vi "BaTS_(Singles).vi"() -> ()   [LabVIEW 2009]
uses:
  <vilib>/Utility/file.llb/Read From Spreadsheet File (DBL).vi
  <vilib>/Utility/miscctls.llb/LVPositionTypeDef.ctl
  <vilib>/Utility/file.llb/Write To Spreadsheet File (I64).vi
  <vilib>/vision/NI_Vision_Development_Module.lvlib
panel:
  out "framesPerSecond":u32
  out "serve to point":dbl[](array[numeric])
  in  "Word._Application":refnum<k7>
  out "p2y":dbl[](array[numeric])
  out "p1y":dbl[](array[numeric])
  out "point frames":dbl[](array[numeric])
  out "service frames":dbl[](array[numeric])
  out "comp_p1 2":dbl[](array[numeric])
  out "comp_p2 2":dbl[](array[numeric])
  out "comp_p2":dbl[](array[numeric])
  out "comp_p1":dbl[](array[numeric])
  out "game":i32[][](array[numeric])
  out "save2_data":dbl[][](array[numeric])
  out "save1_data":dbl[][](array[numeric])
  out "save2":i32[][](array[numeric])
  out "save1":i32[][](array[numeric])
  out "filedata in":dbl[][](array[numeric]) format="%0.3f"
  out "edited\nevents":dbl[][](array[numeric])
  out "edited to play":dbl[](array[numeric])
  out "P2 position":bool
  out "P1 position":bool
  out "p2code":i32
  out "p1code":i32
  out "frames":dbl[](array[numeric])
  out "Events":bool[](array[boolean])
  out "coded data":dbl[][](array[numeric])
  out "frame data":dbl[][](array[numeric])
  out "Score":dbl[][](array[numeric])
  out "OH":bool[](array[boolean])
  out "BH":bool[](array[boolean])
  out "FH":bool[](array[boolean])
  in  "stop":bool
  in  "Tab Control":enum32{"Coding", "Display"}(tab)
  in  "Drag control":u32(slide) min=400 max=3000 scale=0.0..37378.0
  in  "UNDO":bool
  out "Last coded":i32
  in  "Progress...":i32(slide) min=400 max=3000 scale=0.0..36584.0
  in  "1":bool
  in  "E2":bool
  in  "E1":bool
  in  "P2":i32
  in  "W2":bool
  in  "W1":bool
  in  "P1":i32
  in  "Pause 2":bool
  in  "F_Fr":bool
  in  "S_Fr":bool
  out "Video":T1(plugin-control)
  in  "START":bool
  in  "Video file":path caption="Open AVI file"
  in  "Save data":path caption="Save data to file"
  in  "Start Coding":bool
  out "F_frame":u32
  out "S_frame":u32
  in  "playback speed":dbl(slide) step=0.25 scale=0.25..2.0
  in  "fast forward":bool
  in  "TL 2":bool
  in  "BR 2":bool
  in  "BL 2":bool
  in  "BM 2":bool
  in  "CR  2":bool
  in  "CM 2":bool
  in  "CL 2":bool
  in  "TR 2":bool
  in  "TM 2":bool
  in  "TL 3":bool
  in  "BR 3":bool
  in  "BL 3":bool
  in  "BM 3":bool
  in  "CR  3":bool
  in  "CM 3":bool
  in  "CL 3":bool
  in  "TR 3":bool
  in  "TM 3":bool
  in  "Pause 1":bool
  out "coding":i32[][](array[numeric])
  in  "1 6":bool
  in  "2 6":bool
  in  "3 6":bool
  in  "4 6":bool
  in  "5 6":bool
  in  "6 6":bool
  in  "7 6":bool
  in  "8 6":bool
  in  "1 5":bool
  in  "2 5":bool
  in  "3 5":bool
  in  "4 5":bool
  in  "5 5":bool
  in  "6 5":bool
  in  "7 5":bool
  in  "8 5":bool
  in  "8 3":bool
  in  "7 3":bool
  in  "6 3":bool
  in  "5 3":bool
  in  "4 3":bool
  in  "3 3":bool
  in  "2 3":bool
  in  "1 3":bool
  in  "8 4":bool
  in  "7 4":bool
  in  "6 4":bool
  in  "5 4":bool
  in  "4 4":bool
  in  "3 4":bool
  in  "2 4":bool
  in  "1 4":bool
  in  "1 2":bool
  in  "2 2":bool
  in  "3 2":bool
  in  "4 2":bool
  in  "5 2":bool
  in  "6 2":bool
  in  "7 2":bool
  in  "8 2":bool
  in  "5":bool
  in  "6":bool
  in  "7":bool
  in  "8":bool
  in  "1":bool
  in  "2":bool
  in  "3":bool
  in  "4":bool
  in  "S2":bool
  in  "S1":bool
  in  "2":bool
  in  "3":bool
  in  "4":bool
  in  "Pause 3":bool
  in  "court":bool
  in  "Stop and save":bool
  out "Numeric":dbl format="%<%H:%M:%S>t"
  in  "play back":i32(slide)=1 min=0 max=1212 scale=0.0..1212.0
  out "DISP":T1(plugin-control)
  in  "Vid file":path caption="Open AVI file"
  in  "Data file":path caption="Read data from"
  in  "Tab Control 2":enum32{"Edit ", "Data Display", "Momentum"}(tab)
  in  "shots":u8(slide)=2 scale=0.0..5.0
  in  "point 2":bool
  in  "Rally":bool
  in  "Write VI":path caption="Write to AVI file"
  in  "before":u8(slide)=2 scale=5.0..0.0
  in  "Playback Speed":dbl(slide)=1.0 min=0.25 max=30.0 step=0.25 scale=0.25..2.0
  in  "pause":bool
  in  "stop 2":bool
  in  "Playback\nscore":bool
  in  "P2 score":dbl
  in  "P1 score":dbl
  in  "error":bool
  in  "winner":bool
  in  "point 1":bool
  in  "player1":bool
  in  "player2":bool
  in  "1 7":bool
  in  "service2":bool
  in  "service1":bool
  in  "2 7":bool
  in  "3 7":bool
  in  "4 7":bool
  in  "TL":bool
  in  "BR":bool
  in  "BL":bool
  in  "BM":bool
  in  "CR":bool
  in  "CM":bool
  in  "CL":bool
  in  "TR":bool
  in  "TM":bool
  in  "FH 2":bool
  in  "BH 2":bool
  in  "ST":bool
  in  "CR 2":bool
  in  "lob":bool
  in  "clear":bool
  in  "drive":bool
  in  "smash":bool
  in  "defense":bool
  in  "chop":bool
  in  "drop":bool
  in  "net":bool
  in  "OH 2":bool
  in  "Play":bool
  in  "after":u8(slide)=2 scale=0.0..5.0
  in  "write file":bool
  out "Search events":i32(slide) caption="Scaning(events)..." min=400 max=3000 scale=0.0..903.0
  out "Search score":i32(slide) caption="Searching(score)..." min=400 max=3000 scale=0.0..867.0
  out "writing":i32(slide) caption="Writing..." min=400 max=3000 scale=0.0..1212.0
  in  "3 shots":bool
  in  "Compare":bool
  in  "2":string(combo)="1"
  in  "1":string(combo)="1"
  in  "save2":string
  in  "save1":string
  in  "save2":bool
  in  "save1":bool
  in  "Percentage":bool
  in  "display\nselection":string(combo)="1"
  in  "To make white":enum32{""}(tab)
  out "player1 2":string[](array[string])
  out "player2 2":string[](array[string])
  out "P1graph":cluster{dbl[], "array":dbl[]}(graph)={[0.0, nan, 0.0, nan, 0.0, nan, 0.0, nan, 0.0, nan, 0.0, nan, 0.0, nan, 0.0, nan, 0.0], "array"=[1.0, 2.0, 3.0, 4.0, 5.0, 6.0, 7.0, 8.0, 9.0, 10.0, 11.0, 12.0, 13.0, 14.0, 15.0, 16.0, 17.0]}
  out "P2graph":cluster{dbl[], "array":dbl[]}(graph)={[0.0, nan, 0.0, nan, 0.0, nan, 0.0, nan, 0.0, nan, 0.0, nan, 0.0, nan, 0.0, nan, 0.0], "array"=[1.0, 2.0, 3.0, 4.0, 5.0, 6.0, 7.0, 8.0, 9.0, 10.0, 11.0, 12.0, 13.0, 14.0, 15.0, 16.0, 17.0]}
  out "W1/E1":string[](array[string])
  out "W2/E2":string[](array[string])
  out "W/E2":string[](array[string])=["Fore hand", "Back hand", "Over head", "", "Strainght", "Cross", "", "Lob", "Clear", "Drive", "Smash", "Defence", "Chop", "Drop", "Net"]
  out "W/E1":string[](array[string])=["Fore hand", "Back hand", "Over head", "", "Strainght", "Cross", "", "Lob", "Clear", "Drive", "Smash", "Defence", "Chop", "Drop", "Net"]
  out "player2_2":string[](array[string])
  out "player1_2":string[](array[string])
  out "Player 2":string[](array[string])=["Fore hand", "Back hand", "Over head", "", "Straight", "Cross", "", "Smash", "Defense", "Drive/Tap", "Lob", "Drop", "Chop", "Clear", "Net"]
  out "Player 2_2":string[](array[string])=["Fore hand", "Back hand", "Over head", "", "Strainght", "Cross", "", "Lob", "Clear", "Drive", "Smash", "Defence", "Chop", "Drop", "Net"]
  out "Player 1_2":string[](array[string])=["Fore hand", "Back hand", "Over head", "", "Strainght", "Cross", "", "Lob", "Clear", "Drive", "Smash", "Defence", "Chop", "Drop", "Net"]
  out "Player 1":string[](array[string])=["Fore hand", "Back hand", "Over head", "", "Straight", "Cross", "", "Smash", "Defense", "Drive/Tap", "Lob", "Drop", "Chop", "Clear", "Net"]
  out "p2 17":string
  out "p2 16":string
  out "p2 11":string
  out "p2 10":string
  out "p2 9":string
  out "p2 14":string
  out "p2 13":string
  out "p2 12":string
  out "p2 15":string
  out "p1 5":string
  out "p1 7":string
  out "p1 6":string
  out "p1 4":string
  out "p1 1":string
  out "p1 3":string
  out "p1 2":string
  out "p1 8":string
  out "p1 9":string
  in  "to make white 2":enum32{""}(tab)
  out "Shortest rally length(sec)":dbl format="%#_3g"
  out "Longest rally length(sec)":dbl format="%#_3g"
  out "momentum graph":cluster{dbl[], dbl[]}[](graph)
  out "Score":dbl[](array[numeric])
  out "Average rally length(sec)":dbl format="%#_3g"
  out "Rally length(sec)":dbl format="%#_3g"
  in  "edit video":bool
  in  "REPORT":bool
  # "Strategic Analysis Tool for Badminton"
  # "Forehand"
  # "Backhand"
  # "Overhead"
  # "Position"
  # "Straight"
  # "Cross"
  # "Straight"
  # "Cross"
  # "Straight"
  # "Cross"
  # "Smash"
  # "Defence"
  # "Drive/Tap"
  # "Lob"
  # "Drop"
  # "Chop"
  # "Player 2\n\nPlayer 1"
  # "Player 1\n\nPlayer 2"
  # "Clear"
  # "Net"
  # "Score"
  # "© 2012 National Sports Institute of Malaysia All Rights Reserved"
  # "© 2012 National Sports Institute of Malaysia All Rights Reserved"
  # "Shots to Playback"
  # "Score"
  # "Player"
  # "Position"
  # "Special Events"
  # "Playback interval (s)"
  # "to"
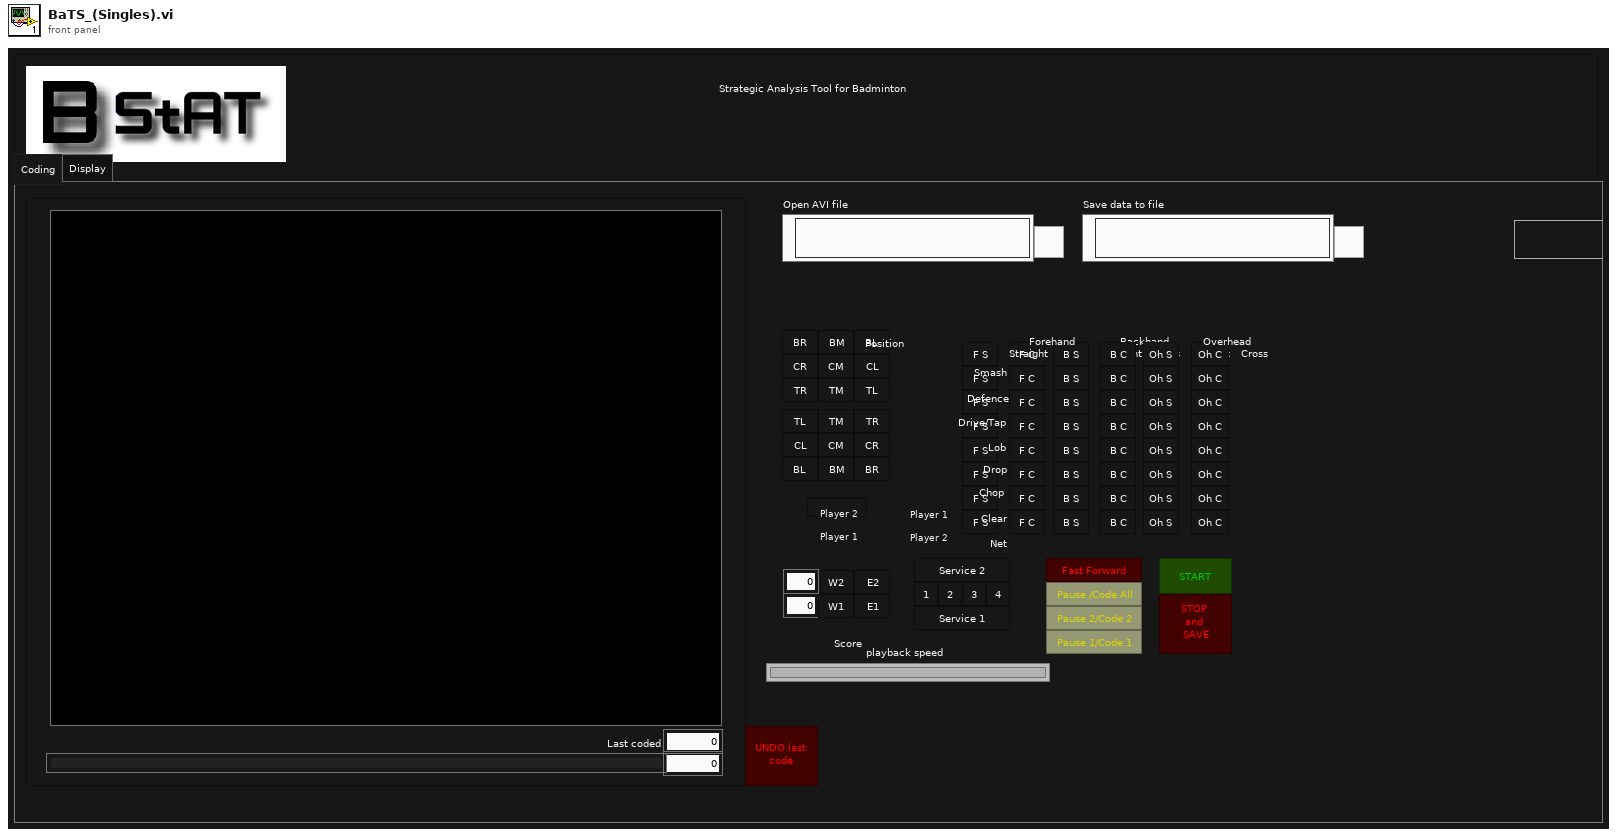
[diagram p1: front panel]
types:
  T1 = typedef "IMAQ Image.ctl" = refnum<image>
  T2 = enum16{"open", "replace", "create", "open or create", "replace or create", "replace or create with confirmation"}
  T3 = typedef "LVPositionTypeDef.ctl" = cluster{"Left":i32, "Top":i32}
  T4 = typedef "Image Type" = u32
  T5 = typedef "AviRefnum.ctl" = refnum<k1>
  T6 = cluster{"width":u32, "height":u32, "framesPerSecond":u32, "compressionFilter":string, "hasData":bool}
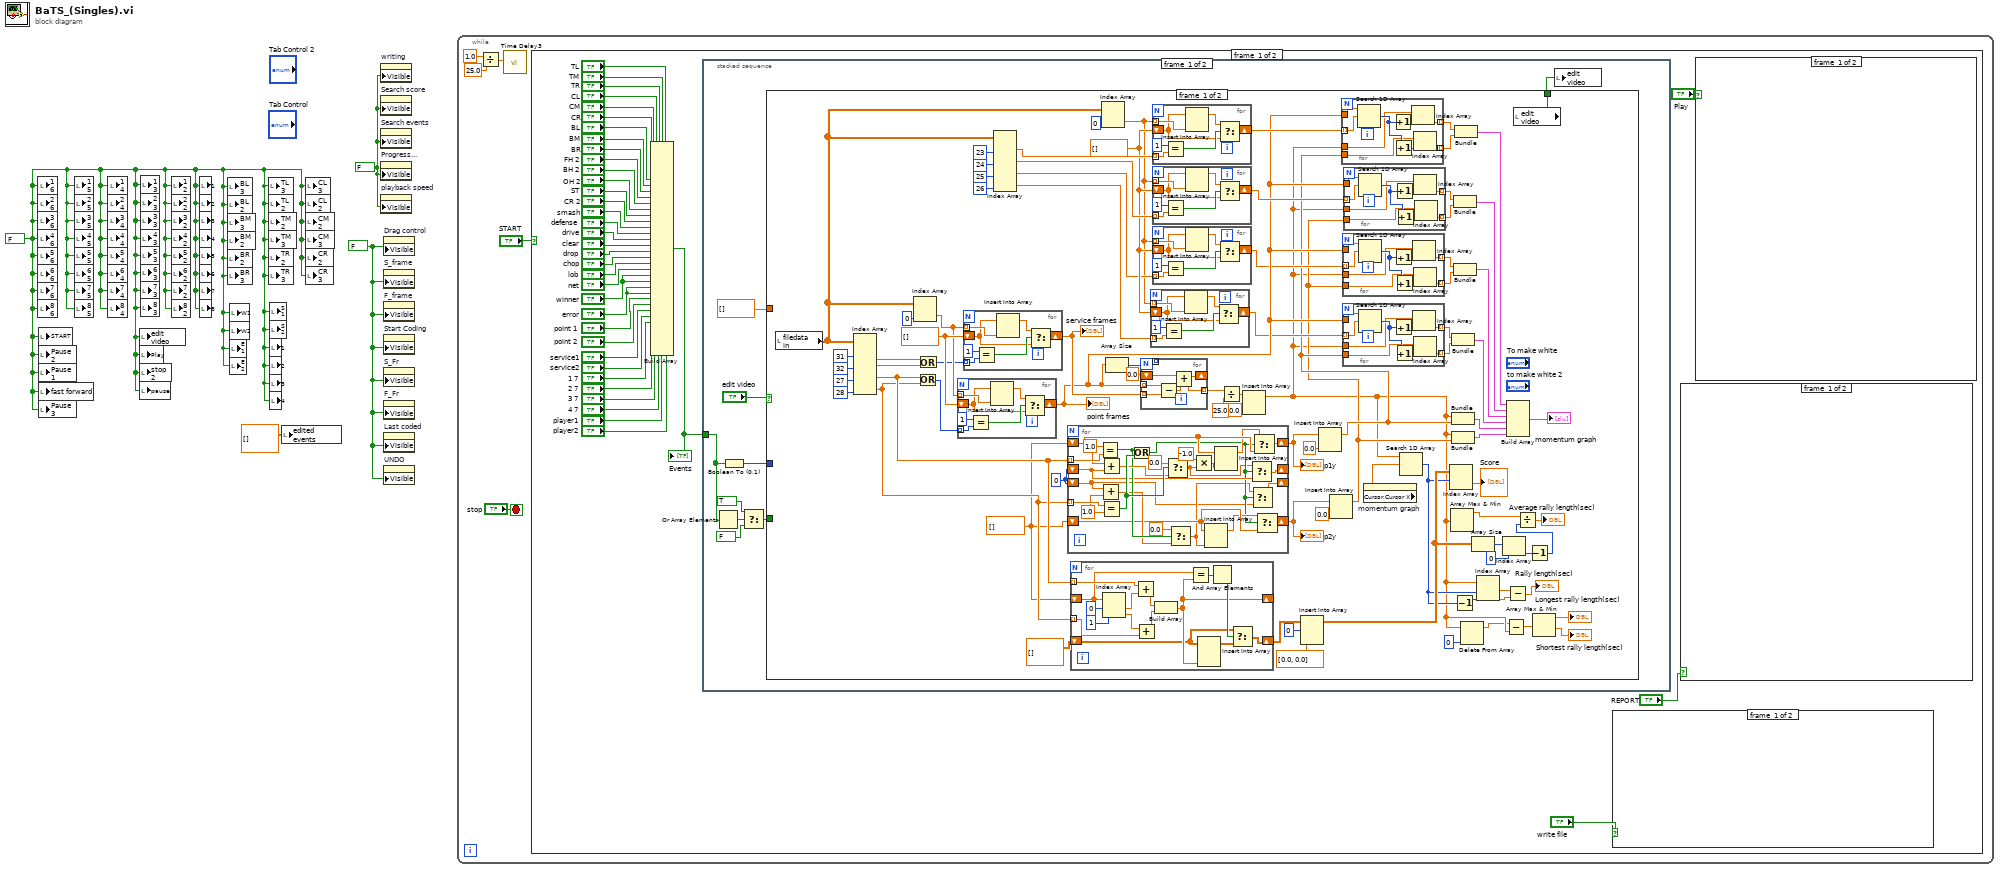
[diagram p0: block diagram]
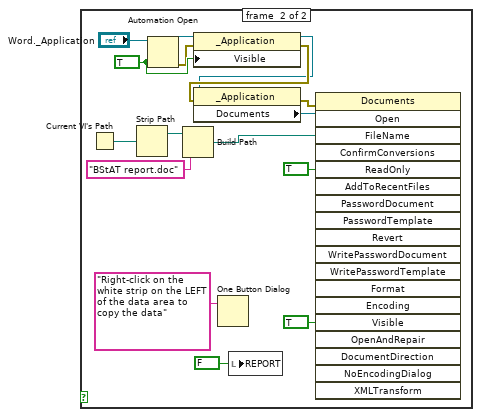
[diagram p2: hidden frame]
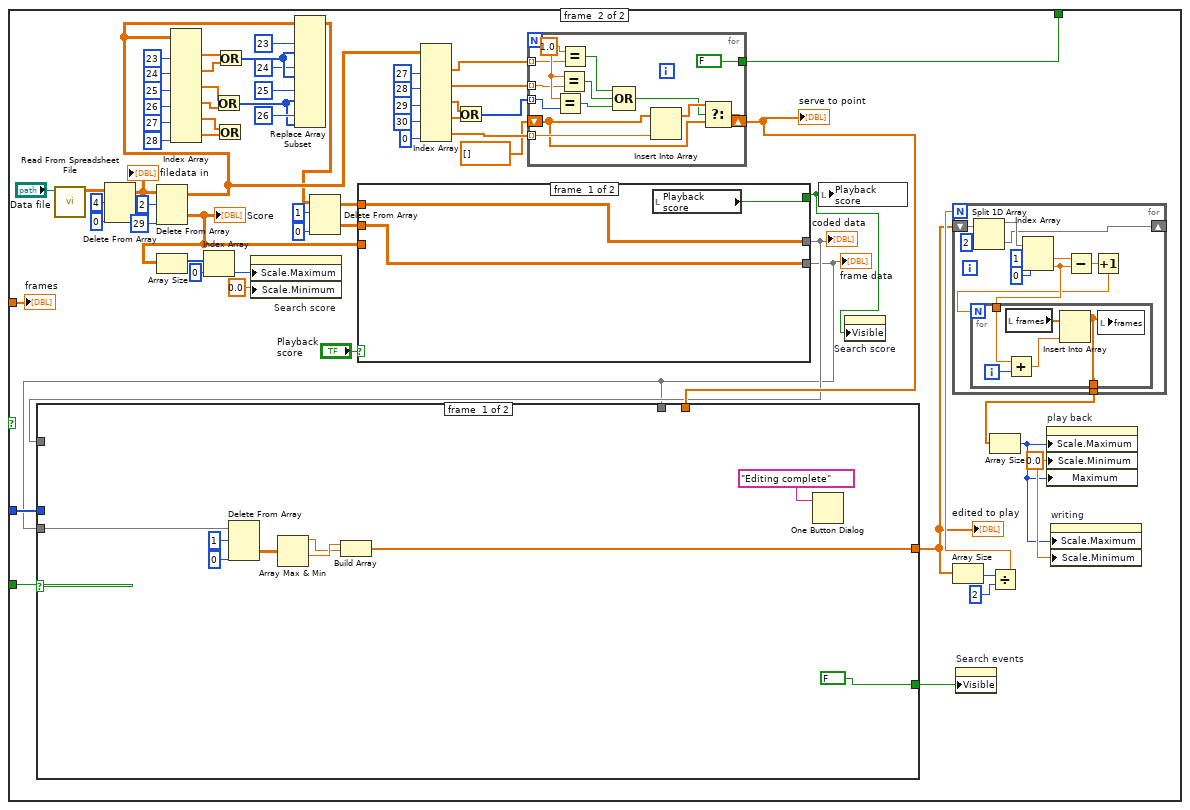
[diagram p3: hidden frame]
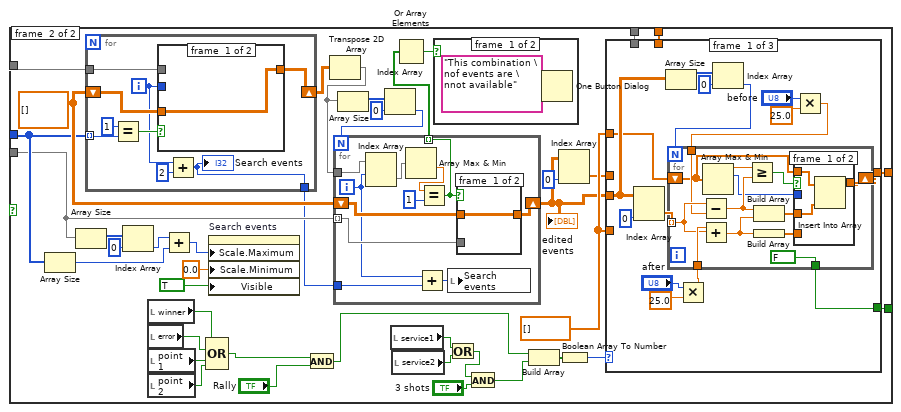
[diagram p4: hidden frame]
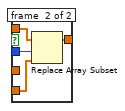
[diagram p5: hidden frame]
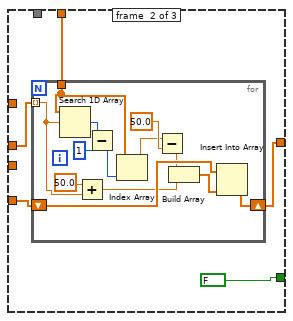
[diagram p6: hidden frame]
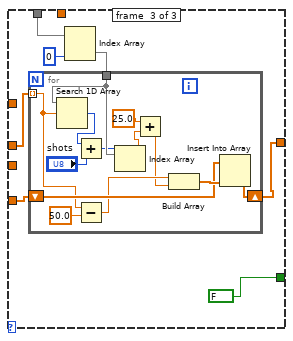
[diagram p7: hidden frame]
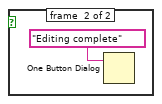
[diagram p8: hidden frame]
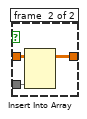
[diagram p9: hidden frame]
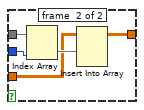
[diagram p10: hidden frame]
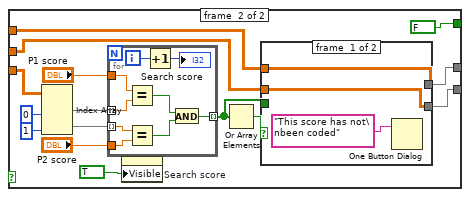
[diagram p11: hidden frame]
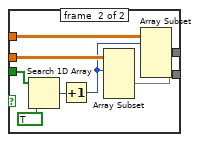
[diagram p12: hidden frame]
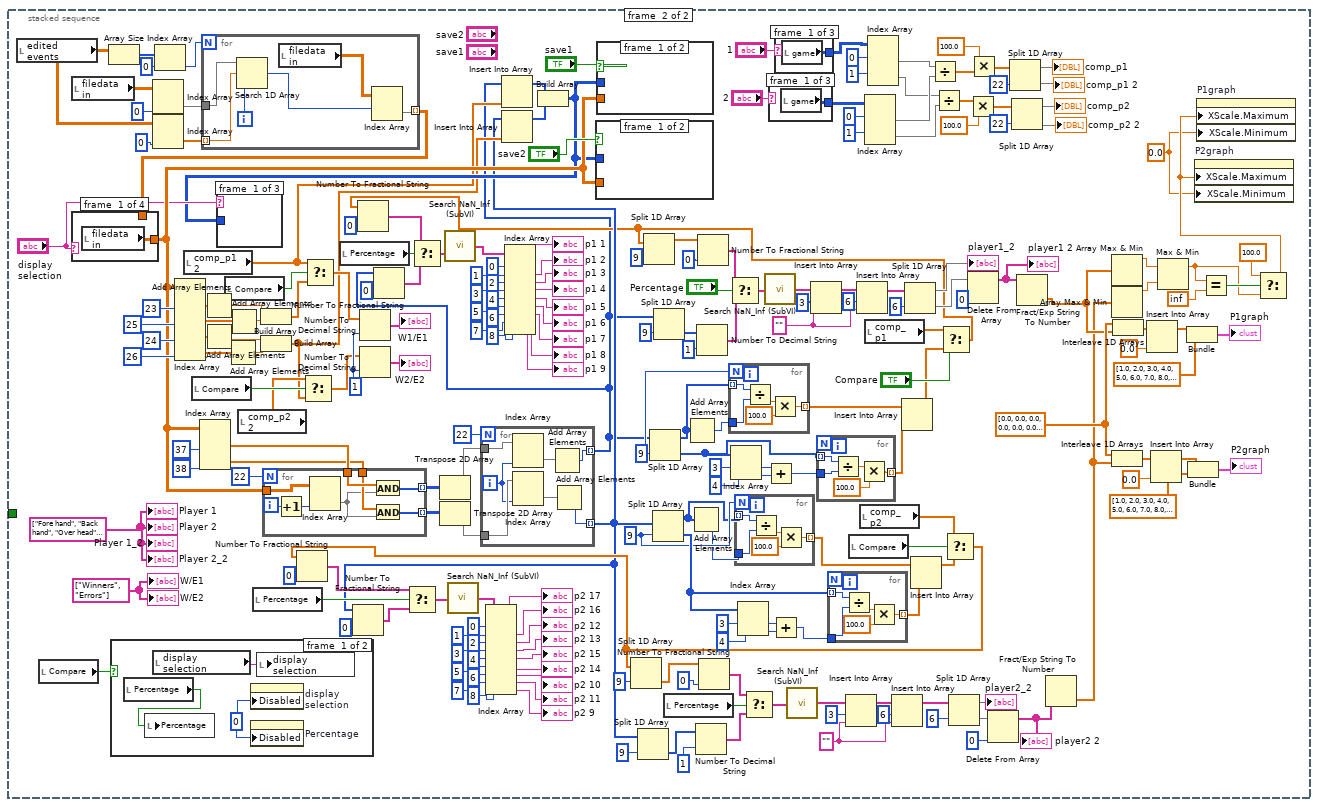
[diagram p13: hidden frame]
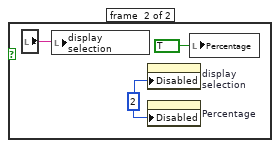
[diagram p14: hidden frame]
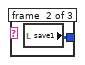
[diagram p15: hidden frame]
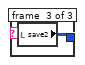
[diagram p16: hidden frame]
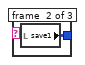
[diagram p17: hidden frame]
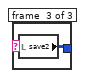
[diagram p18: hidden frame]
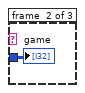
[diagram p19: hidden frame]
diagram:
  w2 = FALSE ("4 6")
  w1 = FALSE ("Visible")
  w3 = FALSE ("Visible")
  n1 = local write "1 6"(w2) -> ()
  n2 = local write "2 6"(w2) -> ()
  n3 = local write "3 6"(w2) -> ()
  n4 = local write "4 6"(w2) -> ()
  n5 = local write "5 6"(w2) -> ()
  n6 = local write "6 6"(w2) -> ()
  n7 = local write "7 6"(w2) -> ()
  n8 = local write "8 6"(w2) -> ()
  n9 = local write "START"(w2) -> ()
  n10 = local write "Pause 2"(w2) -> ()
  n11 = local write "Pause 1"(w2) -> ()
  n12 = local write "fast forward"(w2) -> ()
  n13 = local write "Pause 3"(w2) -> ()
  n14 = local write "1 5"(w2) -> ()
  n15 = local write "2 5"(w2) -> ()
  n16 = local write "3 5"(w2) -> ()
  n17 = local write "4 5"(w2) -> ()
  n18 = local write "5 5"(w2) -> ()
  n19 = local write "6 5"(w2) -> ()
  n20 = local write "7 5"(w2) -> ()
  n21 = local write "8 5"(w2) -> ()
  n22 = local write "1 4"(w2) -> ()
  n23 = local write "2 4"(w2) -> ()
  n24 = local write "3 4"(w2) -> ()
  n25 = local write "4 4"(w2) -> ()
  n26 = local write "5 4"(w2) -> ()
  n27 = local write "6 4"(w2) -> ()
  n28 = local write "7 4"(w2) -> ()
  n29 = local write "8 4"(w2) -> ()
  n30 = local write "edit video"(w2) -> ()
  n31 = local write "Play"(w2) -> ()
  n32 = local write "stop 2"(w2) -> ()
  n33 = local write "pause"(w2) -> ()
  n34 = local write "1 3"(w2) -> ()
  n35 = local write "2 3"(w2) -> ()
  n36 = local write "3 3"(w2) -> ()
  n37 = local write "4 3"(w2) -> ()
  n38 = local write "5 3"(w2) -> ()
  n39 = local write "6 3"(w2) -> ()
  n40 = local write "7 3"(w2) -> ()
  n41 = local write "8 3"(w2) -> ()
  n42 = local write "1 2"(w2) -> ()
  n43 = local write "2 2"(w2) -> ()
  n44 = local write "3 2"(w2) -> ()
  n45 = local write "4 2"(w2) -> ()
  n46 = local write "5 2"(w2) -> ()
  n47 = local write "6 2"(w2) -> ()
  n48 = local write "7 2"(w2) -> ()
  n49 = local write "8 2"(w2) -> ()
  n50 = local write "1"(w2) -> ()
  n51 = local write "2"(w2) -> ()
  n52 = local write "3"(w2) -> ()
  n53 = local write "4"(w2) -> ()
  n54 = local write "5"(w2) -> ()
  n55 = local write "6"(w2) -> ()
  n56 = local write "7"(w2) -> ()
  n57 = local write "8"(w2) -> ()
  n58 = local write "BL 3"(w2) -> ()
  n59 = local write "BL 2"(w2) -> ()
  n60 = local write "BM 3"(w2) -> ()
  n61 = local write "BM 2"(w2) -> ()
  n62 = local write "BR 2"(w2) -> ()
  n63 = local write "BR 3"(w2) -> ()
  n64 = local write "W1"(w2) -> ()
  n65 = local write "W2"(w2) -> ()
  n66 = local write "E1"(w2) -> ()
  n67 = local write "E2"(w2) -> ()
  n68 = local write "TL 3"(w2) -> ()
  n69 = local write "TL 2"(w2) -> ()
  n70 = local write "TM 2"(w2) -> ()
  n71 = local write "TM 3"(w2) -> ()
  n72 = local write "TR 2"(w2) -> ()
  n73 = local write "TR 3"(w2) -> ()
  n74 = local write "S1"(w2) -> ()
  n75 = local write "S2"(w2) -> ()
  n76 = local write "1"(w2) -> ()
  n77 = local write "2"(w2) -> ()
  n78 = local write "3"(w2) -> ()
  n79 = local write "4"(w2) -> ()
  n80 = local write "edited\nevents"(dbl[][] []) -> ()
  n81 = local write "CL 3"(w2) -> ()
  n82 = local write "CL 2"(w2) -> ()
  n83 = local write "CM 2"(w2) -> ()
  n84 = local write "CM 3"(w2) -> ()
  n85 = local write "CR  2"(w2) -> ()
  n86 = local write "CR  3"(w2) -> ()
  n87 = property on="writing" class="Slide (strict)"("Visible"=w3) -> ()  [unwired: 2 in, 2 out]
  n88 = property on="Search score" class="Slide (strict)"("Visible"=w3) -> ()  [unwired: 2 in, 2 out]
  n89 = property on="Search events" class="Slide (strict)"("Visible"=w3) -> ()  [unwired: 2 in, 2 out]
  n90 = property on="Progress..." class="Slide (strict)"("Visible"=w3) -> ()  [unwired: 2 in, 2 out]
  n91 = property on="playback speed" class="Slide (strict)"("Visible"=w3) -> ()  [unwired: 2 in, 2 out]
  n92 = property on="Drag control" class="Slide (strict)"("Visible"=w1) -> ()  [unwired: 2 in, 2 out]
  n93 = property on="S_frame" class="DigNum (strict)"("Visible"=w1) -> ()  [unwired: 2 in, 2 out]
  n94 = property on="F_frame" class="DigNum (strict)"("Visible"=w1) -> ()  [unwired: 2 in, 2 out]
  n95 = property on="Start Coding" class="Bool (strict)"("Visible"=w1) -> ()  [unwired: 2 in, 2 out]
  n96 = property on="S_Fr" class="Bool (strict)"("Visible"=w1) -> ()  [unwired: 2 in, 2 out]
  n97 = property on="F_Fr" class="Bool (strict)"("Visible"=w1) -> ()  [unwired: 2 in, 2 out]
  n98 = property on="Last coded" class="DigNum (strict)"("Visible"=w1) -> ()  [unwired: 2 in, 2 out]
  n99 = property on="UNDO" class="Bool (strict)"("Visible"=w1) -> ()  [unwired: 2 in, 2 out]
  n100 = while {
    stop <- "stop" stop-if-true
    n101 = Divide(x=1.0, y=25.0) -> (x/y=w5:dbl)
    n102 = call "Time Delay3"("Delay Time (s)"=w5) -> ()  [unwired: 10 in, 1 out]
    n103 = case shown="True" "START" {
      frame #0 {
        n104 = Build Array("TL", "TM", "TR", "CL", "CM", "CR", "BL", "BM", "BR", "FH 2", "BH 2", "OH 2", "ST", "CR 2", "smash", "defense", "drive", "clear", "drop", "chop", "lob", "net", "winner", "winner", "error", "error", "point 1", "point 2", "service1", "service2", "1 7", "2 7", "3 7", "4 7", "player1", "player2") -> (w22:bool[])
        "Events" <- w22
        n105 = stacked-sequence {
          tunnel: w22 -> [w69 _]
          frame #0 {
            n106 = Or Array Elements(Boolean array=w69) -> (logical OR=w72:bool)
            n107 = Boolean To (0,1)(Boolean=w69) -> (0, 1=w68:i16[])
            n108 = Select(t=TRUE, s=w72, f=FALSE) -> (s? t:f=w67:bool)
            n109 = case shown="True" "edit video" {
              tunnel: [w157 w287] -> w65
              tunnel: w68 -> [_ w285]
              tunnel: w67 -> [_ w329]
              tunnel: dbl[] [] ("edited\nto play 3") -> [_ w327]
              frame #0 {
                w113 = dbl[] []
                w147 = 0.0 ("new element/subarray")
                w146 = 0.0 ("new element/subarray")
                w145 = 0.0 ("new element/subarray")
                w95 = dbl[] []
                w98 = 0 ("disabled index (col)")
                w138 = dbl[] []
                n110 = local read "filedata in"() -> (w114:dbl[][])
                n111 = Index Array(array=w114, index (col) #1=31 ("length"), index (col) #2=32 ("disabled index (col)"), index (col) #3=27 ("index (col)"), index (col) #4=28 ("index (col)")) -> (element #1=w130:dbl[], element #2=w131:dbl[], element #3=w97:dbl[], element #4=w96:dbl[])  [unwired: 4 in]
                n112 = Index Array(array=w114, index (col)=0 ("disabled index (col)")) -> (element=w137:dbl[])  [unwired: 1 in]
                n113 = Or(x=w97, y=w96) -> (x .or. y?=w136:i32[])
                n114 = Or(x=w130, y=w131) -> (x .or. y?=w133:i32[])
                n115 = for {
                  tunnel: w136 -> [w274] mode=indexing
                  tunnel: w137 -> [w270] mode=indexing
                  shift-right: [w269] -> w109
                  shift-left: w138 -> [w268]
                  n116 = Equal?(x=1, y=w274) -> (x = y?=w272:bool)
                  n117 = Insert Into Array(array=w268, new element=w270) -> (w271:dbl[])  [unwired: 1 in]
                  n118 = Select(t=w271, s=w272, f=w268) -> (s? t:f=w269:dbl[])
                }
                "point frames" <- w109
                n119 = for {
                  tunnel: w133 -> [w281] mode=indexing
                  tunnel: w137 -> [w277] mode=indexing
                  shift-right: [w276] -> w140
                  shift-left: w138 -> [w275]
                  n120 = Equal?(x=1, y=w281) -> (x = y?=w279:bool)
                  n121 = Insert Into Array(array=w275, new element=w277) -> (w278:dbl[])  [unwired: 1 in]
                  n122 = Select(t=w278, s=w279, f=w275) -> (s? t:f=w276:dbl[])
                }
                "service frames" <- w140
                n123 = Index Array(array=w114, index (col) #1=23 ("disabled index (col)"), index (col) #2=24 ("index (col)"), index (col) #3=25 ("index (col)"), index (col) #4=26 ("index (col)")) -> (element #1=w123:dbl[], element #2=w124:dbl[], element #3=w112:dbl[], element #4=w111:dbl[])  [unwired: 4 in]
                n124 = for {
                  shift-right: [w166] -> _
                  shift-left: w98 -> [w165]
                  shift-right: [w162] -> _
                  shift-left: w98 -> [w161]
                  shift-right: [w171] -> w93
                  shift-left: w95 -> [w170]
                  shift-right: [w177] -> w94
                  shift-left: w95 -> [w168]
                  tunnel: w96 -> [w174] mode=indexing
                  tunnel: w97 -> [w182] mode=indexing
                  w173 = 1.0 ("x")
                  w179 = 1.0 ("x")
                  n125 = Equal?(x=w179, y=w182) -> (x = y?=w175:bool)
                  n126 = Add(x=w161, y=w173) -> (x+y=w172:dbl)
                  n127 = Add(x=w179, y=w165) -> (x+y=w178:dbl)
                  n128 = Equal?(x=w174, y=w173) -> (x = y?=w181:bool)
                  n129 = Or(x=w175, y=w181) -> (x .or. y?=w164:bool)
                  n130 = Select(t=0.0, s=w181, f=w178) -> (s? t:f=w158:dbl)
                  n131 = Select(t=0.0, s=w175, f=w172) -> (s? t:f=w163:dbl)
                  n132 = Multiply(x=-1.0 ("y"), y=w158) -> (x*y=w160:dbl)
                  n133 = Insert Into Array(array=w168, new element=w163) -> (w167:dbl[])  [unwired: 1 in]
                  n134 = Insert Into Array(array=w170, new element=w160) -> (w169:dbl[])  [unwired: 1 in]
                  n135 = Select(t=w158, s=w164, f=w165) -> (s? t:f=w166:dbl)
                  n136 = Select(t=w163, s=w164, f=w161) -> (s? t:f=w162:dbl)
                  n137 = Select(t=w169, s=w164, f=w170) -> (s? t:f=w171:dbl[])
                  n138 = Select(t=w167, s=w164, f=w168) -> (s? t:f=w177:dbl[])
                }
                "p1y" <- w93
                "p2y" <- w94
                n139 = for {
                  tunnel: w97 -> [w258] mode=indexing
                  tunnel: w96 -> [w254] mode=indexing
                  shift-right: [w250] -> _
                  shift-left: w95 -> [w253]
                  shift-right: [w248] -> w152
                  shift-left: dbl[][] [] -> [w247]
                  n140 = Index Array(array=w253, index #1=0 ("index"), index #2=1 ("index")) -> (element #1=w259:dbl, element #2=w257:dbl)
                  n141 = Add(x=w258, y=w259) -> (x+y=w256:dbl)
                  n142 = Add(x=w257, y=w254) -> (x+y=w255:dbl)
                  n143 = Build Array(w256, w255) -> (w250:dbl[])
                  n144 = Equal?(x=w253, y=w250) -> (x = y?=w252:bool[])
                  n145 = Insert Into Array(array=w247, new element=w250) -> (w249:dbl[][])  [unwired: 2 in]
                  n146 = And Array Elements(Boolean array=w252) -> (logical AND=w251:bool)
                  n147 = Select(t=w247, s=w251, f=w249) -> (s? t:f=w248:dbl[][])
                }
                n148 = Index Array(array=w114, index (col)=0 ("disabled index (col)")) -> (element=w110:dbl[])  [unwired: 1 in]
                n149 = Array Size(array=w109) -> (size(s)=w139:i32)
                n150 = for {
                  N: w139 -> [w262]
                  tunnel: w109 -> [w267] mode=indexing
                  tunnel: w140 -> [w266] mode=indexing
                  tunnel: [w263] -> w149 mode=indexing
                  shift-right: [w263] -> _
                  shift-left: 0.0 -> [w264]
                  tunnel: [w262] -> _ mode=indexing
                  n151 = Subtract(x=w267, y=w266) -> (x-y=w265:dbl)
                  n152 = Add(x=w264, y=w265) -> (x+y=w263:dbl)
                }
                n153 = for {
                  tunnel: w111 -> [w207] mode=indexing
                  tunnel: w110 -> [w203] mode=indexing
                  shift-right: [w202] -> w107
                  shift-left: w113 -> [w201]
                  n154 = Equal?(x=1, y=w207) -> (x = y?=w205:bool)
                  n155 = Insert Into Array(array=w201, new element=w203) -> (w204:dbl[])  [unwired: 1 in]
                  n156 = Select(t=w204, s=w205, f=w201) -> (s? t:f=w202:dbl[])
                }
                n157 = for {
                  tunnel: w123 -> [w246] mode=indexing
                  tunnel: w110 -> [w242] mode=indexing
                  shift-right: [w241] -> w120
                  shift-left: w113 -> [w240]
                  n158 = Equal?(x=1, y=w246) -> (x = y?=w244:bool)
                  n159 = Insert Into Array(array=w240, new element=w242) -> (w243:dbl[])  [unwired: 1 in]
                  n160 = Select(t=w243, s=w244, f=w240) -> (s? t:f=w241:dbl[])
                }
                n161 = for {
                  tunnel: w124 -> [w239] mode=indexing
                  tunnel: w110 -> [w235] mode=indexing
                  shift-right: [w234] -> w125
                  shift-left: w113 -> [w233]
                  n162 = Equal?(x=1, y=w239) -> (x = y?=w237:bool)
                  n163 = Insert Into Array(array=w233, new element=w235) -> (w236:dbl[])  [unwired: 1 in]
                  n164 = Select(t=w236, s=w237, f=w233) -> (s? t:f=w234:dbl[])
                }
                n165 = for {
                  tunnel: w112 -> [w214] mode=indexing
                  tunnel: w110 -> [w210] mode=indexing
                  shift-right: [w209] -> w108
                  shift-left: w113 -> [w208]
                  n166 = Equal?(x=1, y=w214) -> (x = y?=w212:bool)
                  n167 = Insert Into Array(array=w208, new element=w210) -> (w211:dbl[])  [unwired: 1 in]
                  n168 = Select(t=w211, s=w212, f=w208) -> (s? t:f=w209:dbl[])
                }
                n169 = Divide(x=w149, y=25.0 ("new element/subarray")) -> (x/y=w148:dbl[])
                n170 = Insert Into Array(array=w148, index=w145, new element=w145) -> (w77:dbl[])
                n171 = Insert Into Array(array=w152, index (row)=0, new element=dbl[] [0.0, 0.0] ("new element/subarray")) -> (w90:dbl[][])  [unwired: 1 in]
                n172 = Insert Into Array(array=w93, index=w147, new element=w147) -> (w92:dbl[])
                n173 = Insert Into Array(array=w94, index=w146, new element=w146) -> (w91:dbl[])
                n174 = for {
                  tunnel: w120 -> [w232] mode=indexing
                  tunnel: w109 -> [w231]
                  tunnel: [w229] -> w121 mode=indexing
                  tunnel: [w226] -> w122 mode=indexing
                  tunnel: w77 -> [w225]
                  tunnel: w92 -> [w224]
                  n175 = Search 1D Array(1D array=w231, element=w232) -> (index of element=w227:i32)  [unwired: 1 in]
                  n176 = Increment(x=w227) -> (x+1=w230:i32)
                  n177 = Increment(x=w227) -> (x+1=w228:i32)
                  n178 = Index Array(array=w225, index=w230) -> (element=w229:dbl)
                  n179 = Index Array(array=w224, index=w228) -> (element=w226:dbl)
                }
                n180 = for {
                  tunnel: w108 -> [w200] mode=indexing
                  tunnel: w109 -> [w199]
                  tunnel: [w197] -> w106 mode=indexing
                  tunnel: [w194] -> w105 mode=indexing
                  tunnel: w77 -> [w193]
                  tunnel: w91 -> [w192]
                  n181 = Search 1D Array(1D array=w199, element=w200) -> (index of element=w195:i32)  [unwired: 1 in]
                  n182 = Increment(x=w195) -> (x+1=w198:i32)
                  n183 = Increment(x=w195) -> (x+1=w196:i32)
                  n184 = Index Array(array=w193, index=w198) -> (element=w197:dbl)
                  n185 = Index Array(array=w192, index=w196) -> (element=w194:dbl)
                }
                n186 = for {
                  tunnel: w107 -> [w191] mode=indexing
                  tunnel: w109 -> [w190]
                  tunnel: [w188] -> w104 mode=indexing
                  tunnel: [w185] -> w103 mode=indexing
                  tunnel: w77 -> [w184]
                  tunnel: w92 -> [w183]
                  n187 = Search 1D Array(1D array=w190, element=w191) -> (index of element=w186:i32)  [unwired: 1 in]
                  n188 = Increment(x=w186) -> (x+1=w189:i32)
                  n189 = Increment(x=w186) -> (x+1=w187:i32)
                  n190 = Index Array(array=w184, index=w189) -> (element=w188:dbl)
                  n191 = Index Array(array=w183, index=w187) -> (element=w185:dbl)
                }
                n192 = for {
                  tunnel: w125 -> [w223] mode=indexing
                  tunnel: w109 -> [w222]
                  tunnel: [w220] -> w126 mode=indexing
                  tunnel: [w217] -> w127 mode=indexing
                  tunnel: w77 -> [w216]
                  tunnel: w91 -> [w215]
                  n193 = Search 1D Array(1D array=w222, element=w223) -> (index of element=w218:i32)  [unwired: 1 in]
                  n194 = Increment(x=w218) -> (x+1=w221:i32)
                  n195 = Increment(x=w218) -> (x+1=w219:i32)
                  n196 = Index Array(array=w216, index=w221) -> (element=w220:dbl)
                  n197 = Index Array(array=w215, index=w219) -> (element=w217:dbl)
                }
                n198 = property on="momentum graph" class="XYGraph (strict)"() -> ("Cursor.Cursor X"=w155:dbl)  [unwired: 2 in, 2 out]
                n199 = Search 1D Array(1D array=w77, element=w155) -> (index of element=w82:i32)  [unwired: 1 in]
                n200 = Index Array(array=w90, index (row)=w82) -> (element=→"Score":dbl[])  [unwired: 1 in]
                n201 = Array Max & Min(array=w77) -> (max value=w86:dbl)  [unwired: 3 out]
                n202 = Bundle(w77, w91) -> (w141:cluster{dbl[], dbl[]})  [unwired: 1 in]
                n203 = Bundle(w104, w103) -> (w99:cluster{dbl[], dbl[]})  [unwired: 1 in]
                n204 = Bundle(w77, w92) -> (w142:cluster{dbl[], dbl[]})  [unwired: 1 in]
                n205 = Bundle(w126, w127) -> (w101:cluster{dbl[], dbl[]})  [unwired: 1 in]
                n206 = Bundle(w106, w105) -> (w100:cluster{dbl[], dbl[]})  [unwired: 1 in]
                n207 = Decrement(x=w82) -> (x-1=w83:i32)
                n208 = Bundle(w121, w122) -> (w102:cluster{dbl[], dbl[]})  [unwired: 1 in]
                n209 = Delete From Array(array=w77, index=0) -> (array with subset deleted=w76:dbl[])  [unwired: 1 in, 1 out]
                n210 = Array Size(array=w90) -> (size(s)=w89:i32[])
                n211 = Index Array(array=w77, index #1=w82, index #2=w83) -> (element #1=w80:dbl, element #2=w81:dbl)
                n212 = Index Array(array=w89, index=0) -> (element=w87:i32)
                n213 = Subtract(x=w76, y=w77) -> (x-y=w75:dbl[])
                n214 = Build Array(w102, w101, w100, w99, w142, w141) -> (→"momentum graph":cluster{dbl[], dbl[]}[])
                n215 = Subtract(x=w80, y=w81) -> (x-y=→"Rally length(sec)":dbl)
                n216 = local read "edit video"() -> (w157:bool)
                n217 = Decrement(x=w87) -> (x-1=w85:i32)
                n218 = Divide(x=w86, y=w85) -> (x/y=→"Average rally length(sec)":dbl)
                n219 = Array Max & Min(array=w75) -> (max value=→"Longest rally length(sec)":dbl, min value=→"Shortest rally length(sec)":dbl)  [unwired: 2 out]
              }
              frame #1 {
                w325 = 0.0 ("Scale.Range:Minimum")
                n220 = call-poly <vilib>:"Read From Spreadsheet File.vi"("file path (dialog if empty)"="Data file") -> ("all rows"=w343:dbl[][])  [unwired: 6 in, 4 out]
                n221 = Delete From Array(array=w343, length=4, index (row)=0) -> (array with subset deleted=w322:dbl[][])  [unwired: 1 in, 1 out]
                "filedata in" <- w322
                n222 = Delete From Array(array=w322, length=2, index (col)=29 ("disabled index (col)")) -> (deleted portion=w334:dbl[][], array with subset deleted=w284:dbl[][])  [unwired: 1 in]
                "Score" <- w334
                n223 = Array Size(array=w334) -> (size(s)=w335:i32[])
                n224 = Index Array(array=w284, index (col) #1=23 ("disabled index (col)"), index (col) #2=24 ("index (col)"), index (col) #3=25 ("index (col)"), index (col) #4=26 ("index (col)"), index (col) #5=27 ("index (col)"), index (col) #6=28 ("index (col)")) -> (element #1=w317:dbl[], element #2=w316:dbl[], element #3=w315:dbl[], element #4=w314:dbl[], element #5=w304:dbl[], element #6=w305:dbl[])  [unwired: 6 in]
                n225 = Index Array(array=w335, index=0) -> (element=w333:i32)
                n226 = Or(x=w315, y=w314) -> (x .or. y?=w308:i32[])
                n227 = Or(x=w304, y=w305) -> ()  [unwired: 1 out]
                n228 = Or(x=w317, y=w316) -> (x .or. y?=w313:i32[])
                n229 = property on="Search score" class="Slide (strict)"("Scale.Maximum"=w333, "Scale.Minimum"=0.0 ("Scale.Range:Minimum")) -> ()  [unwired: 2 in, 2 out]
                n230 = Replace Array Subset(array=w284, new element #1=w313, index (col) #1=23 ("disabled index (col)"), new element #2=w313, index (col) #2=24 ("index (col)"), new element #3=w308, index (col) #3=25 ("index (col)"), new element #4=w308, index (col) #4=26 ("index (col)")) -> (w283:dbl[][])  [unwired: 4 in]
                n231 = Delete From Array(array=w283, length=1, index (col)=0 ("disabled index (col)")) -> (deleted portion=w337:dbl[][], array with subset deleted=w338:dbl[][])  [unwired: 1 in]
                n232 = case shown="True" "Playback\nscore" {
                  tunnel: w338 -> [w532 w539]
                  tunnel: w337 -> [w531 w538]
                  tunnel: w334 -> [_ w548]
                  tunnel: [w533 FALSE ("element")] -> w331
                  tunnel: [w531 w536] -> w282
                  tunnel: [w532 w535] -> w288
                  frame #0 {
                    n233 = local read "Playback\nscore"() -> (w533:bool)
                  }
                  frame #1 {
                    n234 = Index Array(array=w548, index (col) #1=0 ("disabled index (col)"), index (col) #2=1 ("index (col)")) -> (element #1=w545:dbl[], element #2=w544:dbl[])  [unwired: 2 in]
                    n235 = for {
                      tunnel: w545 -> [w568] mode=indexing
                      tunnel: w544 -> [w566] mode=indexing
                      tunnel: "P1 score" -> [w567]
                      tunnel: "P2 score" -> [w565]
                      tunnel: [w563] -> w540 mode=indexing
                      i -> [w562]
                      n236 = Equal?(x=w567, y=w568) -> (x = y?=w564:bool)
                      n237 = Equal?(x=w566, y=w565) -> (x = y?=w560:bool)
                      n238 = Increment(x=w562) -> (x+1=→"Search score":i32)
                      n239 = And(x=w564, y=w560) -> (x .and. y?=w563:bool)
                    }
                    n240 = property on="Search score" class="Slide (strict)"("Visible"=TRUE) -> ()  [unwired: 2 in, 2 out]
                    n241 = Or Array Elements(Boolean array=w540) -> (logical OR=w541:bool)
                    n242 = case shown="True" w541 {
                      tunnel: w540 -> [_ w559]
                      tunnel: w539 -> [w551 w557]
                      tunnel: w538 -> [w550 w556]
                      tunnel: [w551 w555] -> w535
                      tunnel: [w550 w554] -> w536
                      frame #0 {
                        n243 = One Button Dialog(message="This score has not\nbeen coded") -> ()  [unwired: 1 in, 1 out]
                      }
                      frame #1 {
                        n244 = Search 1D Array(1D array=w559, element=TRUE) -> (index of element=w553:i32)  [unwired: 1 in]
                        n245 = Increment(x=w553) -> (x+1=w552:i32)
                        n246 = Array Subset(array=w556, index (row)=w552) -> (w554:dbl[][])  [unwired: 3 in]
                        n247 = Array Subset(array=w557, index (row)=w552) -> (w555:dbl[][])  [unwired: 3 in]
                      }
                    }
                  }
                }
                "frame data" <- w282
                "coded data" <- w288
                n248 = Index Array(array=w284, index (col) #1=27 ("disabled index (col)"), index (col) #2=28 ("index (col)"), index (col) #3=29 ("index (col)"), index (col) #4=30 ("index (col)"), index (col) #5=0 ("index (col)")) -> (element #1=w292:dbl[], element #2=w293:dbl[], element #3=w291:dbl[], element #4=w290:dbl[], element #5=w295:dbl[])  [unwired: 5 in]
                n249 = Or(x=w291, y=w290) -> (x .or. y?=w294:i32[])
                n250 = for {
                  tunnel: w292 -> [w350] mode=indexing
                  tunnel: w295 -> [w354] mode=indexing
                  tunnel: w294 -> [w348] mode=indexing
                  tunnel: w293 -> [w349] mode=indexing
                  shift-right: [w356] -> w289
                  shift-left: dbl[] [] -> [w353]
                  tunnel: [FALSE ("edit video")] -> w287
                  w355 = 1.0 ("x")
                  n251 = Equal?(x=w355, y=w348) -> (x = y?=w357:bool)
                  n252 = Equal?(x=w355, y=w349) -> (x = y?=w358:bool)
                  n253 = Equal?(x=w355, y=w350) -> (x = y?=w359:bool)
                  n254 = Compound Arithmetic op=OR(w359, w358, w357) -> (w351:bool)
                  n255 = Insert Into Array(array=w353, new element=w354) -> (w352:dbl[])  [unwired: 1 in]
                  n256 = Select(t=w352, s=w351, f=w353) -> (s? t:f=w356:dbl[])
                }
                "serve to point" <- w289
                n257 = case shown="True" w329 {
                  tunnel: w288 -> [_ w425]
                  tunnel: w285 -> [_ w416]
                  tunnel: w282 -> [w379 w413]
                  tunnel: [w382 w406] -> w302
                  tunnel: [FALSE ("Visible") w405] -> w301
                  tunnel: w289 -> [_ w403]
                  tunnel: w282 -> [_ w399]
                  frame #0 {
                    n258 = Delete From Array(array=w379, length=1, index (col)=0 ("disabled index (col)")) -> (deleted portion=w378:dbl[][])  [unwired: 1 in, 1 out]
                    n259 = Array Max & Min(array=w378) -> (max value=w380:dbl, min value=w381:dbl)  [unwired: 2 out]
                    n260 = Build Array(w381, w380) -> (w382:dbl[])
                    n261 = One Button Dialog(message="Editing complete") -> ()  [unwired: 1 in, 1 out]
                  }
                  frame #1 {
                    w404 = dbl[] []
                    w417 = dbl[][] []
                    n262 = Array Size(array=w416) -> (size(s)=w410:i32)
                    n263 = Array Size(array=w413) -> (size(s)=w414:i32[])
                    n264 = for {
                      tunnel: w416 -> [w524] mode=indexing
                      tunnel: w425 -> [w521]
                      shift-right: [w520] -> w424
                      shift-left: w417 -> [w519]
                      tunnel: [w516] -> w408
                      i -> [w518]
                      n265 = Equal?(x=i16 1, y=w524) -> (x = y?=w522:bool)
                      n266 = case shown="True" w522 {
                        tunnel: w518 -> [_ w530]
                        tunnel: w521 -> [_ w529]
                        tunnel: [w525 w527] -> w520
                        tunnel: w519 -> [w525 w526]
                        frame #0 {
                        }
                        frame #1 {
                          n267 = Index Array(array=w529, index (col)=w530) -> (element=w528:dbl[])  [unwired: 1 in]
                          n268 = Insert Into Array(array=w526, new element=w528) -> (w527:dbl[][])  [unwired: 2 in]
                        }
                      }
                      n269 = Add(x=w518, y=2) -> (x+y=w516:i32)
                      "Search events" <- w516
                    }
                    n270 = Index Array(array=w414, index=0) -> (element=w409:i32)
                    n271 = local read "winner"() -> (w387:bool)
                    n272 = local read "error"() -> (w388:bool)
                    n273 = local read "point 1"() -> (w389:bool)
                    n274 = local read "point 2"() -> (w390:bool)
                    n275 = Add(x=w409, y=w410) -> (x+y=w412:i32)
                    n276 = Compound Arithmetic op=OR(w387, w388, w389, w390) -> (w386:bool)
                    n277 = property on="Search events" class="Slide (strict)"("Scale.Maximum"=w412, "Scale.Minimum"=0.0 ("Scale.Range:Minimum"), "Visible"=TRUE) -> ()  [unwired: 2 in, 2 out]
                    n278 = And(x=w386, y="Rally") -> (x .and. y?=w385:bool)
                    n279 = Transpose 2D Array(2D array=w424) -> (transposed array=w420:dbl[][])
                    n280 = Array Size(array=w420) -> (size(s)=w423:i32[])
                    n281 = Index Array(array=w423, index=0) -> (element=w421:i32)
                    n282 = for {
                      N: w421 -> [_]
                      tunnel: w413 -> [w509] mode=indexing
                      shift-right: [w508] -> w402
                      shift-left: w417 -> [w510]
                      tunnel: w420 -> [w507]
                      tunnel: [w504] -> w419 mode=indexing
                      tunnel: w408 -> [w501]
                      i -> [w502]
                      n283 = Index Array(array=w507, index (row)=w502) -> (element=w506:dbl[])  [unwired: 1 in]
                      n284 = Array Max & Min(array=w506) -> (min value=w505:dbl)  [unwired: 3 out]
                      n285 = Add(x=w502, y=w501) -> (x+y=w503:i32)
                      n286 = Equal?(x=w505, y=1) -> (x = y?=w504:bool)
                      n287 = local write "Search events"(w503) -> ()
                      n288 = case shown="True" w504 {
                        tunnel: w510 -> [w512 w515]
                        tunnel: w509 -> [_ w514]
                        tunnel: [w512 w513] -> w508
                        frame #0 {
                        }
                        frame #1 {
                          n289 = Insert Into Array(array=w515, new element=w514) -> (w513:dbl[][])  [unwired: 2 in]
                        }
                      }
                    }
                    "edited\nevents" <- w402
                    n290 = local read "service1"() -> (w393:bool)
                    n291 = local read "service2"() -> (w394:bool)
                    n292 = Or Array Elements(Boolean array=w419) -> (logical OR=w418:bool)
                    n293 = case shown="True" w418 {
                      frame #0 {
                        n294 = One Button Dialog(message="This combination \nof events are \nnot available") -> ()  [unwired: 1 in, 1 out]
                      }
                      frame #1 {
                        n295 = One Button Dialog(message="Editing complete") -> ()  [unwired: 1 in, 1 out]
                      }
                    }
                    n296 = Or(x=w393, y=w394) -> (x .or. y?=w396:bool)
                    n297 = And(x=w396, y="3 shots") -> (x .and. y?=w392:bool)
                    n298 = Build Array(w385, w392) -> (w398:bool[])
                    n299 = Index Array(array=w402, index (col)=0 ("disabled index (col)")) -> (element=w400:dbl[])  [unwired: 1 in]
                    n300 = Boolean Array To Number(Boolean array=w398) -> (number=w397:u32)
                    n301 = case shown="0, Default" w397 {
                      tunnel: w402 -> [w429 _ _]
                      tunnel: [w428 w463 w479] -> w406
                      tunnel: [w427 FALSE ("Visible") FALSE ("Visible")] -> w405
                      tunnel: w404 -> [w426 _ _]
                      tunnel: w404 -> [_ w465 w483]
                      tunnel: w403 -> [_ w464 _]
                      tunnel: w400 -> [_ w461 w484]
                      tunnel: w399 -> [_ _ w482]
                      frame #0 {
                        n302 = Index Array(array=w429, index (col)=0 ("disabled index (col)")) -> (element=w431:dbl[])  [unwired: 1 in]
                        n303 = Array Size(array=w429) -> (size(s)=w435:i32[])
                        n304 = Multiply(x="after", y=25.0) -> (x*y=w433:dbl)
                        n305 = Index Array(array=w435, index=0) -> (element=w430:i32)
                        n306 = Multiply(x="before", y=25.0) -> (x*y=w434:dbl)
                        n307 = for {
                          N: w430 -> [_]
                          tunnel: w434 -> [w451]
                          tunnel: w433 -> [w453]
                          tunnel: w431 -> [w452] mode=indexing
                          shift-right: [w443] -> w428
                          shift-left: w426 -> [w447]
                          tunnel: [FALSE ("Visible")] -> w427
                          n308 = Subtract(x=w452, y=w451) -> (x-y=w449:dbl)
                          n309 = Add(x=w453, y=w452) -> (x+y=w448:dbl)
                          n310 = Array Max & Min(array=w447) -> (max value=w450:dbl, max index (indices)=w445:i32)  [unwired: 2 out]
                          n311 = Greater Or Equal?(x=w450, y=w449) -> (x >= y?=w446:bool)
                          n312 = Build Array(w449, w448) -> (w442:dbl[])
                          n313 = Build Array(w448) -> (w444:dbl[])
                          n314 = case shown="True" w446 {
                            tunnel: w447 -> [w456 w460]
                            tunnel: w445 -> [_ w459]
                            tunnel: w444 -> [_ w458]
                            tunnel: [w455 w457] -> w443
                            tunnel: w442 -> [w454 _]
                            frame #0 {
                              n315 = Insert Into Array(array=w456, new element=w454) -> (w455:dbl[])  [unwired: 1 in]
                            }
                            frame #1 {
                              n316 = Replace Array Subset(array=w460, new element=w458, index=w459) -> (w457:dbl[])
                            }
                          }
                        }
                      }
                      frame #1 {
                        n317 = for {
                          tunnel: w461 -> [w466] mode=indexing
                          shift-right: [w473] -> w463
                          shift-left: w465 -> [w474]
                          tunnel: w464 -> [w467]
                          n318 = Search 1D Array(1D array=w467, element=w466) -> (index of element=w478:i32)  [unwired: 1 in]
                          n319 = Add(x=50.0, y=w466) -> (x+y=w471:dbl)
                          n320 = Subtract(x=w478, y=1) -> (x-y=w476:i32)
                          n321 = Index Array(array=w467, index=w476) -> (element=w468:dbl)
                          n322 = Subtract(x=w468, y=50.0 ("x")) -> (x-y=w472:dbl)
                          n323 = Build Array(w472, w471) -> (w475:dbl[])
                          n324 = Insert Into Array(array=w474, new element=w475) -> (w473:dbl[])  [unwired: 1 in]
                        }
                      }
                      frame #2 {
                        n325 = Index Array(array=w482, index (col)=0 ("disabled index (col)")) -> (element=w480:dbl[])  [unwired: 1 in]
                        n326 = for {
                          tunnel: w484 -> [w488] mode=indexing
                          shift-right: [w496] -> w479
                          shift-left: w483 -> [w497]
                          tunnel: w480 -> [w491]
                          n327 = Search 1D Array(1D array=w491, element=w488) -> (index of element=w490:i32)  [unwired: 1 in]
                          n328 = Add(x=w490, y="shots") -> (x+y=w489:i32)
                          n329 = Subtract(x=w488, y=50.0 ("x")) -> (x-y=w495:dbl)
                          n330 = Index Array(array=w491, index=w489) -> (element=w487:dbl)
                          n331 = Add(x=25.0, y=w487) -> (x+y=w494:dbl)
                          n332 = Build Array(w495, w494) -> (w498:dbl[])
                          n333 = Insert Into Array(array=w497, new element=w498) -> (w496:dbl[])  [unwired: 1 in]
                        }
                      }
                    }
                  }
                }
                "edited to play" <- w302
                n334 = local write "Playback\nscore"(w331) -> ()
                n335 = property on="Search score" class="Slide (strict)"("Visible"=w331) -> ()  [unwired: 2 in, 2 out]
                n336 = Array Size(array=w302) -> (size(s)=w328:i32)
                n337 = property on="Search events" class="Slide (strict)"("Visible"=w301) -> ()  [unwired: 2 in, 2 out]
                n338 = Divide(x=w328, y=2) -> (x/y=w324:dbl)
                n339 = for {
                  N: w324 -> [_]
                  shift-right: [w364] -> _
                  shift-left: w302 -> [w366]
                  tunnel: [w360] -> w326
                  n340 = Split 1D Array(array=w366, index=2) -> (first subarray=w365:dbl[], second subarray=w364:dbl[])
                  n341 = Index Array(array=w365, index #1=1 ("index"), index #2=0 ("index")) -> (element #1=w370:dbl, element #2=w363:dbl)
                  n342 = Subtract(x=w370, y=w363) -> (x-y=w362:dbl)
                  n343 = Increment(x=w362) -> (x+1=w361:dbl)
                  n344 = for {
                    N: w361 -> [_]
                    tunnel: w363 -> [w375]
                    tunnel: [w371] -> w360
                    i -> [w374]
                    n345 = local read "frames"() -> (w373:dbl[])
                    n346 = Add(x=w375, y=w374) -> (x+y=w372:dbl)
                    n347 = Insert Into Array(array=w373, new element=w372) -> (w371:dbl[])  [unwired: 1 in]
                    n348 = local write "frames"(w371) -> ()
                  }
                }
                n349 = Array Size(array=w326) -> (size(s)=w323:i32)
                n350 = property on="play back" class="Slide (strict)"("Scale.Maximum"=w323, "Scale.Minimum"=w325, "Maximum"=w323) -> ()  [unwired: 2 in, 2 out]
                n351 = property on="writing" class="Slide (strict)"("Scale.Maximum"=w323, "Scale.Minimum"=w325) -> ()  [unwired: 2 in, 2 out]
                "frames" <- w327
              }
            }
            n352 = local write "edit video"(w65) -> ()
          }
          frame #1 {
            w608 = 0.0 ("X Scale.Range:Minimum")
            w647 = i16 1 ("width (-)")
            w790 = dbl[] [0.0, 0.0, 0.0, 0.0, 0.0, 0.0, 0.0, 0.0] ("array")
            w776 = string[] ["Winners", "Errors"] ("W/E1")
            w757 = string[] ["Fore hand", "Back hand", "Over head", "", "Straight", "Cross", "", "Smash", "Defence", "Drive/Tap", "Lob", "Drop", "Chop", "Clear", "Net"] ("Player 2")
            w751 = "" ("new element/subarray")
            w750 = "" ("new element/subarray")
            w702 = 9 ("index")
            w697 = 9 ("index")
            n353 = local read "edited\nevents"() -> (w668:dbl[][])
            n354 = local read "Compare"() -> (w624:bool)
            n355 = local read "filedata in"() -> (w674:dbl[][])
            n356 = Array Size(array=w668) -> (size(s)=w680:i32[])
            n357 = case shown="False" w624 {
              frame #0 {
                w791 = u8 0 ("Disabled")
                n358 = local read "Percentage"() -> (w792:bool)
                n359 = local write "Percentage"(w792) -> ()
                n360 = local read "display\nselection"() -> (w793:string)
                n361 = property on="display\nselection" class="CmbBox"("Disabled"=w791) -> ()  [unwired: 2 in, 2 out]
                n362 = property on="Percentage" class="Bool (strict)"("Disabled"=w791) -> ()  [unwired: 2 in, 2 out]
                n363 = local write "display\nselection"(w793) -> ()
              }
              frame #1 {
                w794 = u8 2 ("Disabled")
                n364 = local read "1"() -> (w796:string)
                n365 = local write "display\nselection"(w796) -> ()
                n366 = property on="display\nselection" class="CmbBox"("Disabled"=w794) -> ()  [unwired: 2 in, 2 out]
                n367 = property on="Percentage" class="Bool (strict)"("Disabled"=w794) -> ()  [unwired: 2 in, 2 out]
                n368 = local write "Percentage"(TRUE ("t")) -> ()
              }
            }
            n369 = Index Array(array=w674, index (col)=0 ("disabled index (col)")) -> (element=w676:dbl[])  [unwired: 1 in]
            n370 = Index Array(array=w668, index (col)=0 ("disabled index (col)")) -> (element=w673:dbl[])  [unwired: 1 in]
            n371 = Index Array(array=w680, index=0) -> (element=w678:i32)
            n372 = local read "comp_p1 2"() -> (w622:dbl[])
            n373 = local read "Compare"() -> (w631:bool)
            n374 = for {
              N: w678 -> [_]
              tunnel: w676 -> [w818]
              tunnel: w673 -> [w817] mode=indexing
              tunnel: [w814] -> w666 mode=indexing
              i -> [w819]
              n375 = Search 1D Array(1D array=w818, element=w817, start index (0)=w819) -> (index of element=w815:i32)
              n376 = local read "filedata in"() -> (w816:dbl[][])
              n377 = Index Array(array=w816, index (row)=w815) -> (element=w814:dbl[])  [unwired: 1 in]
            }
            n378 = case shown="\"1\", Default" "display\nselection" {
              tunnel: [w804 w805 w806 w807] -> w667
              tunnel: w666 -> [_ w805 _ _]
              frame #0 {
                n379 = local read "filedata in"() -> (w804:dbl[][])
              }
              frame #1 {
              }
              frame #2 {
                n380 = local read "save1_data"() -> (w806:dbl[][])
              }
              frame #3 {
                n381 = local read "save2_data"() -> (w807:dbl[][])
              }
            }
            n382 = Index Array(array=w667, index (col) #1=23 ("disabled index (col)"), index (col) #2=25 ("index (col)"), index (col) #3=24 ("index (col)"), index (col) #4=26 ("index (col)")) -> (element #1=w759:dbl[], element #2=w764:dbl[], element #3=w765:dbl[], element #4=w763:dbl[])  [unwired: 4 in]
            n383 = Index Array(array=w667, index (col) #1=37 ("disabled index (col)"), index (col) #2=38 ("index (col)")) -> (element #1=w687:dbl[], element #2=w684:dbl[])  [unwired: 2 in]
            n384 = Add Array Elements(numeric array=w759) -> (sum=w779:dbl)
            n385 = Add Array Elements(numeric array=w765) -> (sum=w778:dbl)
            n386 = local read "Compare"() -> (w634:bool)
            n387 = Add Array Elements(numeric array=w763) -> (sum=w777:dbl)
            n388 = Add Array Elements(numeric array=w764) -> (sum=w780:dbl)
            n389 = local read "comp_p2 2"() -> (w630:dbl[])
            n390 = local read "Percentage"() -> (w755:bool)
            n391 = Build Array(w779, w780) -> (w633:dbl[])
            n392 = Build Array(w778, w777) -> (w623:dbl[])
            n393 = for {
              N: 22 -> [_]
              tunnel: w667 -> [w854]
              tunnel: w687 -> [w853]
              tunnel: w684 -> [w852]
              tunnel: [w850] -> w685 mode=indexing
              tunnel: [w849] -> w686 mode=indexing
              i -> [w847]
              n394 = Increment(x=w847) -> (x+1=w848:i32)
              n395 = Index Array(array=w854, index (col)=w848) -> (element=w851:dbl[])  [unwired: 1 in]
              n396 = And(x=w853, y=w851) -> (x .and. y?=w850:i32[])
              n397 = And(x=w852, y=w851) -> (x .and. y?=w849:i32[])
            }
            n398 = Select(t=w630, s=w631, f=w623) -> (s? t:f=w629:dbl[])
            n399 = Select(t=w622, s=w634, f=w633) -> (s? t:f=w632:dbl[])
            n400 = local read "Percentage"() -> (w756:bool)
            n401 = Number To Decimal String(number=w632, width (-)=w647) -> (decimal integer string=→"W1/E1":string[])
            n402 = Number To Decimal String(number=w629, width (-)=w647) -> (decimal integer string=→"W2/E2":string[])
            n403 = Transpose 2D Array(2D array=w685) -> (transposed array=w696:i32[][])
            n404 = Transpose 2D Array(2D array=w686) -> (transposed array=w695:i32[][])
            n405 = for {
              N: 22 -> [_]
              tunnel: w696 -> [w846]
              tunnel: w695 -> [w845]
              tunnel: [w842] -> w580 mode=indexing
              tunnel: [w841] -> w587 mode=indexing
              i -> [w844]
              n406 = Index Array(array=w846, index (col)=w844) -> (element=w843:i32[])  [unwired: 1 in]
              n407 = Index Array(array=w845, index (col)=w844) -> (element=w840:i32[])  [unwired: 1 in]
              n408 = Add Array Elements(numeric array=w843) -> (sum=w842:i32)
              n409 = Add Array Elements(numeric array=w840) -> (sum=w841:i32)
            }
            n410 = Number To Fractional String(number=w587, precision (6)=i16 0) -> (F-format string=w586:string[])  [unwired: 2 in]
            n411 = Number To Fractional String(number=w580, precision (6)=i16 0) -> (F-format string=w582:string[])  [unwired: 2 in]
            n412 = Insert Into Array(array=w580, new element=w622) -> (w672:i32[])  [unwired: 1 in]
            n413 = Insert Into Array(array=w587, new element=w623) -> (w671:i32[])  [unwired: 1 in]
            n414 = Build Array(w672, w671) -> (w664:i32[][])
            n415 = case shown="\"0\", Default" "display\nselection" {
              tunnel: w664 -> [_ w803 _]
              frame #0 {
              }
              frame #1 {
                "game" <- w803
              }
              frame #2 {
              }
            }
            n416 = case shown="False" "save2" {
              tunnel: w664 -> [_ w810]
              tunnel: w667 -> [_ w808]
              frame #0 {
              }
              frame #1 {
                n417 = local write "save2"(FALSE ("save2")) -> ()
                "save2" <- w810
                "save2_data" <- w808
              }
            }
            n418 = case shown="False" "save1" {
              tunnel: w664 -> [_ w813]
              tunnel: w667 -> [_ w811]
              frame #0 {
              }
              frame #1 {
                n419 = local write "save1"(FALSE ("save1")) -> ()
                "save1" <- w813
                "save1_data" <- w811
              }
            }
            n420 = Split 1D Array(array=w587, index=9) -> (second subarray=w739:i32[])  [unwired: 1 out]
            n421 = Split 1D Array(array=w580, index=w697) -> (first subarray=w698:i32[], second subarray=w708:i32[])
            n422 = Split 1D Array(array=w587, index=w702) -> (first subarray=w701:i32[], second subarray=w706:i32[])
            n423 = Split 1D Array(array=w580, index=9) -> (second subarray=w733:i32[])  [unwired: 1 out]
            n424 = local read "Percentage"() -> (w743:bool)
            n425 = Add Array Elements(numeric array=w698) -> (sum=w699:i32)
            n426 = Add Array Elements(numeric array=w701) -> (sum=w700:i32)
            n427 = Number To Decimal String(number=w739, width (-)=i16 1 ("precision (6)")) -> (decimal integer string=w745:string[])
            n428 = Number To Decimal String(number=w733, width (-)=i16 1 ("precision (6)")) -> (decimal integer string=w742:string[])
            n429 = for {
              N: w697 -> [_]
              tunnel: w698 -> [w839] mode=indexing
              tunnel: w699 -> [w838]
              tunnel: [w835] -> w728 mode=indexing
              n430 = Divide(x=w839, y=w838) -> (x/y=w837:dbl)
              n431 = Multiply(x=w837, y=100.0) -> (x*y=w835:dbl)
            }
            n432 = Index Array(array=w708, index #1=3 ("index"), index #2=4 ("index")) -> (element #1=w703:i32, element #2=w704:i32)
            n433 = for {
              N: w702 -> [_]
              tunnel: w701 -> [w834] mode=indexing
              tunnel: w700 -> [w833]
              tunnel: [w830] -> w626 mode=indexing
              n434 = Divide(x=w834, y=w833) -> (x/y=w832:dbl)
              n435 = Multiply(x=w832, y=100.0) -> (x*y=w830:dbl)
            }
            n436 = Index Array(array=w706, index #1=3 ("index"), index #2=4 ("index")) -> (element #1=w694:i32, element #2=w693:i32)
            n437 = Add(x=w703, y=w704) -> (x+y=w707:i32)
            n438 = case shown="\"4\"" "2" {
              tunnel: [w797 w798 w799] -> w656
              frame #0 {
                n439 = local read "game"() -> (w797:i32[][])
              }
              frame #1 {
                n440 = local read "save1"() -> (w798:i32[][])
              }
              frame #2 {
                n441 = local read "save2"() -> (w799:i32[][])
              }
            }
            n442 = Add(x=w694, y=w693) -> (x+y=w705:i32)
            n443 = case shown="\"1\", Default" "1" {
              tunnel: [w800 w801 w802] -> w660
              frame #0 {
                n444 = local read "game"() -> (w800:i32[][])
              }
              frame #1 {
                n445 = local read "save1"() -> (w801:i32[][])
              }
              frame #2 {
                n446 = local read "save2"() -> (w802:i32[][])
              }
            }
            n447 = for {
              tunnel: w708 -> [w824] mode=indexing
              tunnel: w707 -> [w823]
              tunnel: [w820] -> w729 mode=indexing
              n448 = Divide(x=w824, y=w823) -> (x/y=w822:dbl)
              n449 = Multiply(x=w822, y=100.0) -> (x*y=w820:dbl)
            }
            n450 = for {
              tunnel: w706 -> [w829] mode=indexing
              tunnel: w705 -> [w828]
              tunnel: [w825] -> w730 mode=indexing
              n451 = Divide(x=w829, y=w828) -> (x/y=w827:dbl)
              n452 = Multiply(x=w827, y=100.0) -> (x*y=w825:dbl)
            }
            n453 = local read "Compare"() -> (w637:bool)
            n454 = local read "comp_p2"() -> (w638:dbl[])
            n455 = Index Array(array=w656, index (row) #1=0 ("index (row)"), index (row) #2=1 ("index (row)")) -> (element #1=w654:i32[], element #2=w652:i32[])  [unwired: 2 in]
            n456 = local read "comp_p1"() -> (w639:dbl[])
            n457 = Index Array(array=w660, index (row) #1=0 ("index (row)"), index (row) #2=1 ("index (row)")) -> (element #1=w655:i32[], element #2=w653:i32[])  [unwired: 2 in]
            n458 = Insert Into Array(array=w728, new element=w729) -> (w627:dbl[])  [unwired: 1 in]
            n459 = Insert Into Array(array=w626, new element=w730) -> (w625:dbl[])  [unwired: 1 in]
            n460 = Divide(x=w655, y=w654) -> (x/y=w649:dbl[])
            n461 = Divide(x=w653, y=w652) -> (x/y=w648:dbl[])
            n462 = Select(t=w639, s="Compare", f=w627) -> (s? t:f=w584:dbl[])
            n463 = Number To Fractional String(number=w584, precision (6)=i16 0) -> (F-format string=w581:string[])  [unwired: 2 in]
            n464 = Select(t=w581, s=w756, f=w582) -> (s? t:f=w570:string[])
            n465 = call "Search NaN_Inf (SubVI).vi"("in"=w570) -> ("out"=w569:string[])
            n466 = Index Array(array=w569, index #1=0 ("index"), index #2=1 ("index"), index #3=2 ("index"), index #4=3 ("index"), index #5=4 ("index"), index #6=5 ("index"), index #7=6 ("index"), index #8=7 ("index"), index #9=8 ("index")) -> (element #1=→"p1 1":string, element #2=→"p1 2":string, element #3=→"p1 3":string, element #4=→"p1 4":string, element #5=→"p1 5":string, element #6=→"p1 6":string, element #7=→"p1 7":string, element #8=→"p1 8":string, element #9=→"p1 9":string)
            n467 = Split 1D Array(array=w584, index=9) -> (second subarray=w735:dbl[])  [unwired: 1 out]
            n468 = Number To Fractional String(number=w735, precision (6)=i16 0) -> (F-format string=w741:string[])  [unwired: 2 in]
            n469 = Select(t=w741, s="Percentage", f=w742) -> (s? t:f=w607:string[])
            n470 = call "Search NaN_Inf (SubVI).vi"("in"=w607) -> ("out"=w606:string[])
            n471 = Insert Into Array(array=w606, index=3, new element=w750) -> (w748:string[])
            n472 = Insert Into Array(array=w748, index=6, new element=w750) -> (w766:string[])
            n473 = Split 1D Array(array=w766, index=6) -> (first subarray=→"player1_2":string[], second subarray=w769:string[])
            n474 = Select(t=w638, s=w637, f=w625) -> (s? t:f=w590:dbl[])
            n475 = Number To Fractional String(number=w590, precision (6)=i16 0) -> (F-format string=w589:string[])  [unwired: 2 in]
            n476 = Select(t=w589, s=w755, f=w586) -> (s? t:f=w591:string[])
            n477 = call "Search NaN_Inf (SubVI).vi"("in"=w591) -> ("out"=w594:string[])
            n478 = Index Array(array=w594, index #1=0 ("index"), index #2=1 ("index"), index #3=2 ("index"), index #4=3 ("index"), index #5=4 ("index"), index #6=5 ("index"), index #7=6 ("index"), index #8=7 ("index"), index #9=8 ("index")) -> (element #1=→"p2 17":string, element #2=→"p2 16":string, element #3=→"p2 12":string, element #4=→"p2 13":string, element #5=→"p2 15":string, element #6=→"p2 14":string, element #7=→"p2 10":string, element #8=→"p2 11":string, element #9=→"p2 9":string)
            n479 = Split 1D Array(array=w590, index=9) -> (second subarray=w736:dbl[])  [unwired: 1 out]
            n480 = Number To Fractional String(number=w736, precision (6)=i16 0) -> (F-format string=w744:string[])  [unwired: 2 in]
            n481 = Select(t=w744, s=w743, f=w745) -> (s? t:f=w604:string[])
            n482 = call "Search NaN_Inf (SubVI).vi"("in"=w604) -> ("out"=w605:string[])
            n483 = Insert Into Array(array=w605, index=3, new element=w751) -> (w753:string[])
            n484 = Insert Into Array(array=w753, index=6, new element=w751) -> (w774:string[])
            n485 = Split 1D Array(array=w774, index=6) -> (first subarray=→"player2_2":string[], second subarray=w772:string[])
            n486 = Multiply(x=w648, y=100.0 ("new element/subarray")) -> (x*y=w643:dbl[])
            n487 = Delete From Array(array=w769, index=0) -> (array with subset deleted=w609:string[])  [unwired: 1 in, 1 out]
            "player1 2" <- w609
            n488 = Multiply(x=100.0 ("new element/subarray"), y=w649) -> (x*y=w646:dbl[])
            n489 = Delete From Array(array=w772, index=0) -> (array with subset deleted=w610:string[])  [unwired: 1 in, 1 out]
            "player2 2" <- w610
            n490 = Split 1D Array(array=w646, index=22) -> (first subarray=→"comp_p1":dbl[], second subarray=→"comp_p1 2":dbl[])
            n491 = Split 1D Array(array=w643, index=22) -> (first subarray=→"comp_p2":dbl[], second subarray=→"comp_p2 2":dbl[])
            n492 = Fract/Exp String To Number(string=w609) -> (number=w603:dbl[])  [unwired: 3 in, 1 out]
            n493 = Fract/Exp String To Number(string=w610) -> (number=w602:dbl[])  [unwired: 3 in, 1 out]
            n494 = Array Max & Min(array=w603) -> (max value=w618:dbl)  [unwired: 3 out]
            n495 = Array Max & Min(array=w602) -> (max value=w617:dbl)  [unwired: 3 out]
            n496 = Interleave 1D Arrays(w790, w602) -> (w619:dbl[])
            n497 = Interleave 1D Arrays(w790, w603) -> (w621:dbl[])
            n498 = Insert Into Array(array=w621, new element=0.0 ("new element/subarray")) -> (w784:dbl[])  [unwired: 1 in]
            n499 = Insert Into Array(array=w619, new element=0.0 ("new element/subarray")) -> (w785:dbl[])  [unwired: 1 in]
            n500 = Max & Min(x=w618, y=w617) -> (max(x,y)=w612:dbl)  [unwired: 1 out]
            n501 = Bundle(w784, "array"=dbl[] [1.0, 2.0, 3.0, 4.0, 5.0, 6.0, 7.0, 8.0, 9.0, 10.0, 11.0, 12.0, 13.0, 14.0, 15.0, 16.0, 17.0]) -> (→"P1graph":cluster{dbl[], "array":dbl[]})  [unwired: 1 in]
            n502 = Bundle(w785, "array"=dbl[] [1.0, 2.0, 3.0, 4.0, 5.0, 6.0, 7.0, 8.0, 9.0, 10.0, 11.0, 12.0, 13.0, 14.0, 15.0, 16.0, 17.0]) -> (→"P2graph":cluster{dbl[], "array":dbl[]})  [unwired: 1 in]
            n503 = Equal?(x=w612, y=inf) -> (x = y?=w614:bool)
            n504 = Select(t=100.0, s=w614, f=w612) -> (s? t:f=w611:dbl)
            n505 = property on="P2graph" class="XYGraph (strict)"("XScale.Maximum"=w611, "XScale.Minimum"=w608) -> ()  [unwired: 2 in, 2 out]
            n506 = property on="P1graph" class="XYGraph (strict)"("XScale.Maximum"=w611, "XScale.Minimum"=w608) -> ()  [unwired: 2 in, 2 out]
            "Player 1" <- w757
            "Player 1_2" <- w757
            "Player 2_2" <- w757
            "Player 2" <- w757
            "W/E1" <- w776
            "W/E2" <- w776
          }
        }
        n507 = case shown="True" "write file" {
          frame #0 {
          }
          frame #1 {
            w867 = T4 4 items=["Grayscale (U8)", "Grayscale (I16)", "Grayscale (SGL)", "Complex (CSG)", "RGB (U32)", "HSL (U32)", "RGB (U64)"] ("Image Type")
            n508 = local write "writing"(0 ("writing")) -> ()
            n509 = property on="writing" class="Slide (strict)"("Visible"=TRUE) -> ()  [unwired: 2 in, 2 out]
            n510 = local read "Vid file"() -> (w869:path)
            n511 = call "IMAQ AVI Create"("Compression Filter"="Microsoft Video 1", "Frames Per Second"=u32 25, "AVI Path"="Write VI") -> ("Avi Refnum"=w870:T5)  [unwired: 7 in, 1 out]
            n512 = local read "frames"() -> (w872:dbl[])
            n513 = call "IMAQ Create"("Image Name"="write", "Image Type"=w867) -> ("New Image"=w865:T1, "error out"=w864:errorcluster)  [unwired: 3 in]
            n514 = call "IMAQ AVI Open"("AVI Path"=w869) -> ("Avi Refnum"=w868:T5)  [unwired: 9 in, 1 out]
            n515 = Array Size(array=w872) -> (size(s)=w871:i32)
            n516 = for {
              N: w871 -> [_]
              tunnel: w870 -> [w880]
              tunnel: w868 -> [w876]
              tunnel: w865 -> [w882]
              tunnel: w864 -> [w881]
              tunnel: [w880] -> w863
              tunnel: [FALSE ("Play")] -> w861
              tunnel: ["Writing complete" ("message")] -> w860
              tunnel: [w876] -> w858
              tunnel: [w875] -> w857
              i -> [w878]
              n517 = local read "frames"() -> (w884:dbl[])
              n518 = Index Array(array=w884, index=w878) -> (element=w883:dbl)
              n519 = call "IMAQ AVI Read Frame"("error in (no error)"=w881, "Frame Number"=w883, "Image"=w882, "Avi Refnum"=w876) -> ("error out"=w885:errorcluster, "Image Out"=w875:T1)  [unwired: 4 in, 2 out]
              n520 = call "IMAQ AVI Write Frame"("error in (no error)"=w885, "Image"=w875, "Avi Refnum"=w880) -> ()  [unwired: 7 in, 2 out]
              "writing" <- w878
            }
            n521 = local write "write file"(w861) -> ()
            n522 = property on="writing" class="Slide (strict)"("Visible"=w861) -> ()  [unwired: 2 in, 2 out]
            n523 = call "IMAQ AVI Close"("Avi Refnum"=w858) -> ("error out"=w856:errorcluster)  [unwired: 10 in]
            n524 = One Button Dialog(message=w860) -> ()  [unwired: 1 in, 1 out]
            n525 = call "IMAQ AVI Close"("Avi Refnum"=w863) -> ()  [unwired: 10 in, 1 out]
            n526 = call "IMAQ Dispose"("Image"=w857, "error in (no error)"=w856) -> ()  [unwired: 4 in, 1 out]
          }
        }
        n527 = case shown="False" "REPORT" {
          frame #0 {
          }
          frame #1 {
            w63 = TRUE ("open new instance (false)")
            n528 = Current VI's Path() -> (path=w61:path)
            n529 = Strip Path(path=w61) -> (stripped path=w62:path)  [unwired: 1 out]
            n530 = Automation Open(Automation Refnum="Word._Application", 9:w63) -> (Automation Refnum=w54:refnum<k7>, error out=w55:errorcluster)  [unwired: 2 in]
            n531 = Build Path(base path=w62, name or relative path="BStAT report.doc") -> (appended path=w48:path)
            n532 = property class="_Application"(reference=w54, error in=w55, "Visible"=w63) -> (reference out=w56:refnum<k7>, error out=w57:errorcluster)
            n533 = property class="_Application"(reference=w56, error in=w57) -> (error out=w59:errorcluster, "Documents"=w58:refnum<k7>)  [unwired: 1 out]
            n534 = One Button Dialog(message="Right-click on the white strip on the LEFT of the data area to copy the data") -> ()  [unwired: 1 in, 1 out]
            n535 = local write "REPORT"(FALSE ("REPORT")) -> ()
            n536 = invoke class="Documents" method="Open"(reference=w58, error in=w59, "FileName"=w48, "ReadOnly"=TRUE, "Visible"=TRUE) -> ()  [unwired: 14 in, 19 out]
          }
        }
        n537 = case shown="True" "Play" {
          frame #0 {
          }
          frame #1 {
            w897 = T4 4 items=["Grayscale (U8)", "Grayscale (I16)", "Grayscale (SGL)", "Complex (CSG)", "RGB (U32)", "HSL (U32)", "RGB (U64)"] ("Image Type")
            w898 = T4 4 items=["Grayscale (U8)", "Grayscale (I16)", "Grayscale (SGL)", "Complex (CSG)", "RGB (U32)", "HSL (U32)", "RGB (U64)"] ("Image Type")
            n538 = local write "play back"(0 ("play back")) -> ()
            n539 = call "IMAQ AVI Open"("AVI Path"="Vid file") -> ("Avi Refnum"=w890:T5)  [unwired: 9 in, 1 out]
            n540 = call "IMAQ Create"("Image Name"="Disp1", "Image Type"=w898) -> ("New Image"=w894:T1, "error out"=w893:errorcluster)  [unwired: 3 in]
            n541 = call "IMAQ Create"("Image Name"="Disp2", "Image Type"=w897) -> ("New Image"=w892:T1, "error out"=w891:errorcluster)  [unwired: 3 in]
            n542 = while {
              tunnel: w890 -> [w920]
              tunnel: w894 -> [w924]
              tunnel: w893 -> [w923]
              tunnel: w892 -> [w922]
              tunnel: w891 -> [w921]
              tunnel: [FALSE ("Play")] -> w886
              tunnel: [w920] -> w888
              stop <- w909 stop-if-true
              n543 = while {
                stop <- w926 continue-if-true
                n544 = local read "stop 2"() -> (w925:bool)
                n545 = Not(x=w925) -> (.not. x?=w928:bool)
                n546 = And(x=w928, y="pause") -> (x .and. y?=w926:bool)
              }
              n547 = local read "frames"() -> (w914:dbl[])
              n548 = Increment(x="play back") -> (x+1=w905:i32)
              n549 = Array Max & Min(array=w914) -> (max value=w912:dbl)  [unwired: 3 out]
              n550 = Index Array(array=w914, index=w905) -> (element=w913:dbl)
              n551 = call "IMAQ AVI Read Frame"("error in (no error)"=w923, "Frame Number"=w913, "Image"=w924, "Avi Refnum"=w920) -> ("Image Out"=w919:T1)  [unwired: 4 in, 3 out]
              n552 = call "IMAQ Resample"("X Resolution"=680, "Y Resolution"=520, "error in (no error)"=w921, "Image Dst"=w922, "Image Src"=w919) -> ("Image Dst Out"=→"DISP":T1)  [unwired: 5 in, 1 out]
              n553 = Divide(x=w905, y=25.0) -> (x/y=→"Numeric":dbl)
              n554 = Multiply(x="Playback Speed", y=25.0) -> (x*y=w904:dbl)
              n555 = local write "play back"(w905) -> ()
              n556 = Divide(x=1.0, y=w904) -> (x/y=w901:dbl)
              n557 = Equal?(x=w913, y=w912) -> (x = y?=w911:bool)
              n558 = Or(x=w911, y="stop 2") -> (x .or. y?=w909:bool)
              n559 = call "play delay"("Delay Time (s)"=w901) -> ()  [unwired: 10 in, 1 out]
            }
            n560 = local write "Play"(FALSE ("Play")) -> ()
            n561 = call "IMAQ AVI Close"("Avi Refnum"=w888) -> ()  [unwired: 10 in, 1 out]
            n562 = local write "stop 2"(w886) -> ()
          }
        }
      }
      frame #1 {
        w929 = u32 0 ("S_frame")
        n563 = local write "Drag control"(w929) -> ()
        n564 = local write "START"(FALSE ("START")) -> ()
        n565 = stacked-sequence {
          frame #0 {
            w934 = T4 4 items=["Grayscale (U8)", "Grayscale (I16)", "Grayscale (SGL)", "Complex (CSG)", "RGB (U32)", "HSL (U32)", "RGB (U64)"] ("Image Type")
            w940 = 0 ("p2code")
            w948 = T4 4 items=["Grayscale (U8)", "Grayscale (I16)", "Grayscale (SGL)", "Complex (CSG)", "RGB (U32)", "HSL (U32)", "RGB (U64)"] ("Image Type")
            n566 = call "IMAQ Create"("Image Name"="setup1", "Image Type"=w934) -> ("New Image"=w932:T1, "error out"=w931:errorcluster)  [unwired: 3 in]
            n567 = call "IMAQ Create"("Image Name"="setup", "Image Type"=w948) -> ("New Image"=w946:T1, "error out"=w944:errorcluster)  [unwired: 3 in]
            n568 = call "IMAQ AVI Open"("AVI Path"="Video file") -> ("Avi Refnum"=w949:T5)  [unwired: 9 in, 1 out]
            n569 = call "IMAQ AVI Get Info"("Avi Refnum"=w949) -> ("Number of Frames"=w950:u32, "Avi Refnum (duplicate)"=w942:T5, "Frame Data"=w936:T6)  [unwired: 6 in, 2 out]
            n570 = while {
              tunnel: w942 -> [w966]
              tunnel: w946 -> [w965]
              tunnel: w944 -> [w964]
              tunnel: [FALSE ("Visible")] -> w937
              tunnel: [w961] -> w945
              tunnel: [w960] -> w941
              tunnel: w932 -> [w953]
              tunnel: w931 -> [w952]
              stop <- "Start Coding" stop-if-true
              w959 = TRUE ("Visible")
              n571 = while {
                tunnel: "Drag control" -> [w972]
                stop <- w970 stop-if-true
                n572 = local read "Drag control"() -> (w967:u32)
                n573 = Not Equal?(x=w972, y=w967) -> (x != y?=w969:bool)
                n574 = case shown="True" "F_Fr" {
                  tunnel: w972 -> [_ w975]
                  frame #0 {
                  }
                  frame #1 {
                    n575 = local write "F_frame"(w975) -> ()
                    n576 = local write "F_Fr"(FALSE ("F_Fr")) -> ()
                  }
                }
                n577 = case shown="True" "S_Fr" {
                  tunnel: w972 -> [_ w977]
                  frame #0 {
                  }
                  frame #1 {
                    n578 = local write "S_frame"(w977) -> ()
                    n579 = local write "S_Fr"(FALSE ("S_Fr")) -> ()
                  }
                }
                n580 = local read "Start Coding"() -> (w968:bool)
                n581 = Or(x=w969, y=w968) -> (x .or. y?=w970:bool)
              }
              n582 = call "IMAQ AVI Read Frame"("error in (no error)"=w964, "Frame Number"="Drag control", "Image"=w965, "Avi Refnum"=w966) -> ("Image Out"=w955:T1, "Avi Refnum (duplicate)"=w961:T5)  [unwired: 4 in, 2 out]
              n583 = call "IMAQ Resample"("X Resolution"=680, "Y Resolution"=520, "error in (no error)"=w952, "Image Dst"=w953, "Image Src"=w955) -> ("Image Dst Out"=→"Video":T1)  [unwired: 5 in, 1 out]
              n584 = property on="Drag control" class="Slide (strict)"("Visible"=w959) -> ()  [unwired: 2 in, 2 out]
              n585 = property on="S_frame" class="DigNum (strict)"("Visible"=w959) -> ()  [unwired: 2 in, 2 out]
              n586 = property on="Start Coding" class="Bool (strict)"("Visible"=w959) -> ()  [unwired: 2 in, 2 out]
              n587 = property on="S_Fr" class="Bool (strict)"("Visible"=w959) -> ()  [unwired: 2 in, 2 out]
              n588 = property on="F_frame" class="DigNum (strict)"("Visible"=w959) -> ()  [unwired: 2 in, 2 out]
              n589 = property on="F_Fr" class="Bool (strict)"("Visible"=w959) -> ()  [unwired: 2 in, 2 out]
              n590 = local read "S_frame"() -> (w960:u32)
            }
            n591 = Decrement(x=w950) -> (x-1=w939:u32)
            n592 = property on="Drag control" class="Slide (strict)"("Scale.Maximum"=w939, "Scale.Minimum"=0.0 ("Scale.Range:Minimum")) -> ()  [unwired: 2 in, 2 out]
            n593 = Unbundle By Name(w936) -> ("framesPerSecond"=→"framesPerSecond":u32)
            n594 = call "IMAQ AVI Close"("Avi Refnum"=w945) -> ()  [unwired: 10 in, 1 out]
            n595 = local write "p2code"(w940) -> ()
            n596 = local write "p1code"(w940) -> ()
            n597 = property on="S_frame" class="DigNum (strict)"("Visible"=w937) -> ()  [unwired: 2 in, 2 out]
            n598 = property on="F_frame" class="DigNum (strict)"("Visible"=w937) -> ()  [unwired: 2 in, 2 out]
            n599 = property on="Start Coding" class="Bool (strict)"("Visible"=w937) -> ()  [unwired: 2 in, 2 out]
            n600 = property on="S_Fr" class="Bool (strict)"("Visible"=w937) -> ()  [unwired: 2 in, 2 out]
            n601 = property on="F_Fr" class="Bool (strict)"("Visible"=w937) -> ()  [unwired: 2 in, 2 out]
            n602 = local write "Start Coding"(w937) -> ()
            n603 = local write "Progress..."(w941) -> ()
            n604 = One Button Dialog(message="Please Select the start and end points\nof the video for coding ") -> ()  [unwired: 1 in, 1 out]
          }
          frame #1 {
            w980 = T4 4 items=["Grayscale (U8)", "Grayscale (I16)", "Grayscale (SGL)", "Complex (CSG)", "RGB (U32)", "HSL (U32)", "RGB (U64)"] ("Image Type")
            w991 = "\r"
            w987 = TRUE ("Visible")
            w985 = TRUE ("Visible")
            w1006 = T4 4 items=["Grayscale (U8)", "Grayscale (I16)", "Grayscale (SGL)", "Complex (CSG)", "RGB (U32)", "HSL (U32)", "RGB (U64)"] ("Image Type")
            n605 = local read "Video file"() -> (w995:path)
            n606 = call "IMAQ Create"("Image Name"="code", "Image Type"=w1006) -> ("New Image"=w1005:T1, "error out"=w1004:errorcluster)  [unwired: 3 in]
            n607 = call "IMAQ Create"("Image Name"="code 2", "Image Type"=w980) -> ("New Image"=w978:T1, "error out"=w979:errorcluster)  [unwired: 3 in]
            n608 = call "IMAQ AVI Open"("AVI Path"=w995) -> ("Avi Refnum"=w1003:T5)  [unwired: 9 in, 1 out]
            n609 = while {
              tunnel: w1005 -> [w1042]
              tunnel: w1004 -> [w1041]
              tunnel: w1003 -> [w1048]
              tunnel: [FALSE] -> w988
              tunnel: [w1050] -> w984
              tunnel: [w1047] -> w989
              tunnel: [w1033] -> w983
              tunnel: [w1032] -> w982
              tunnel: w979 -> [w1020]
              tunnel: w978 -> [w1019]
              stop <- w1026 stop-if-true
              n610 = case shown="True" "court" {
                frame #0 {
                  n611 = property on="P2" class="DigNum (strict)"("Position"=T3 {"Left"=805, "Top"=395} ("Position 3")) -> ()  [unwired: 2 in, 2 out]
                  n612 = property on="P1" class="DigNum (strict)"("Position"=T3 {"Left"=805, "Top"=419} ("Position 4")) -> ()  [unwired: 2 in, 2 out]
                  n613 = property on="E2" class="Bool (strict)"("Position"=T3 {"Left"=876, "Top"=396} ("Position 28")) -> ()  [unwired: 2 in, 2 out]
                  n614 = property on="E1" class="Bool (strict)"("Position"=T3 {"Left"=876, "Top"=420} ("Position 27")) -> ()  [unwired: 2 in, 2 out]
                  n615 = property on="W1" class="Bool (strict)"("Position"=T3 {"Left"=840, "Top"=420} ("Position 19")) -> ()  [unwired: 2 in, 2 out]
                  n616 = property on="W2" class="Bool (strict)"("Position"=T3 {"Left"=840, "Top"=396} ("Position 20")) -> ()  [unwired: 2 in, 2 out]
                  n617 = property on="Pause 2" class="Bool (strict)"("Position"=T3 {"Left"=1068, "Top"=432}) -> ()  [unwired: 2 in, 2 out]
                  n618 = property on="Pause 1" class="Bool (strict)"("Position"=T3 {"Left"=1068, "Top"=456} ("Position 2")) -> ()  [unwired: 2 in, 2 out]
                  n619 = property on="TL 3" class="Bool (strict)"("Position"=T3 {"Left"=804, "Top"=235} ("Position 5")) -> ()  [unwired: 2 in, 2 out]
                  n620 = property on="TL 2" class="Bool (strict)"("Position"=T3 {"Left"=876, "Top"=204} ("Position 6")) -> ()  [unwired: 2 in, 2 out]
                  n621 = property on="CL 3" class="Bool (strict)"("Position"=T3 {"Left"=804, "Top"=259} ("Position 7")) -> ()  [unwired: 2 in, 2 out]
                  n622 = property on="CL 2" class="Bool (strict)"("Position"=T3 {"Left"=876, "Top"=180} ("Position 8")) -> ()  [unwired: 2 in, 2 out]
                  n623 = property on="BL 3" class="Bool (strict)"("Position"=T3 {"Left"=804, "Top"=283} ("Position 9")) -> ()  [unwired: 2 in, 2 out]
                  n624 = property on="BL 2" class="Bool (strict)"("Position"=T3 {"Left"=876, "Top"=156} ("Position 10")) -> ()  [unwired: 2 in, 2 out]
                  n625 = property on="S1" class="Bool (strict)"("Position"=T3 {"Left"=936, "Top"=432} ("Position 11")) -> ()  [unwired: 2 in, 2 out]
                  n626 = property on="S2" class="Bool (strict)"("Position"=T3 {"Left"=936, "Top"=384} ("Position 12")) -> ()  [unwired: 2 in, 2 out]
                  n627 = property on="TM 3" class="Bool (strict)"("Position"=T3 {"Left"=840, "Top"=235} ("Position 13")) -> ()  [unwired: 2 in, 2 out]
                  n628 = property on="TM 2" class="Bool (strict)"("Position"=T3 {"Left"=840, "Top"=204} ("Position 14")) -> ()  [unwired: 2 in, 2 out]
                  n629 = property on="CM 3" class="Bool (strict)"("Position"=T3 {"Left"=840, "Top"=259} ("Position 15")) -> ()  [unwired: 2 in, 2 out]
                  n630 = property on="CM 2" class="Bool (strict)"("Position"=T3 {"Left"=840, "Top"=180} ("Position 16")) -> ()  [unwired: 2 in, 2 out]
                  n631 = property on="BM 3" class="Bool (strict)"("Position"=T3 {"Left"=840, "Top"=283} ("Position 17")) -> ()  [unwired: 2 in, 2 out]
                  n632 = property on="BM 2" class="Bool (strict)"("Position"=T3 {"Left"=840, "Top"=156} ("Position 18")) -> ()  [unwired: 2 in, 2 out]
                  n633 = property on="TR 3" class="Bool (strict)"("Position"=T3 {"Left"=876, "Top"=235} ("Position 21")) -> ()  [unwired: 2 in, 2 out]
                  n634 = property on="TR 2" class="Bool (strict)"("Position"=T3 {"Left"=804, "Top"=204} ("Position 22")) -> ()  [unwired: 2 in, 2 out]
                  n635 = property on="CR  3" class="Bool (strict)"("Position"=T3 {"Left"=876, "Top"=259} ("Position 23")) -> ()  [unwired: 2 in, 2 out]
                  n636 = property on="CR  2" class="Bool (strict)"("Position"=T3 {"Left"=804, "Top"=180} ("Position 24")) -> ()  [unwired: 2 in, 2 out]
                  n637 = property on="BR 3" class="Bool (strict)"("Position"=T3 {"Left"=876, "Top"=283} ("Position 25")) -> ()  [unwired: 2 in, 2 out]
                  n638 = property on="BR 2" class="Bool (strict)"("Position"=T3 {"Left"=804, "Top"=156} ("Position 26")) -> ()  [unwired: 2 in, 2 out]
                }
                frame #1 {
                  n639 = property on="P2" class="DigNum (strict)"("Position"=T3 {"Left"=805, "Top"=419} ("Position 3")) -> ()  [unwired: 2 in, 2 out]
                  n640 = property on="P1" class="DigNum (strict)"("Position"=T3 {"Left"=805, "Top"=395} ("Position 4")) -> ()  [unwired: 2 in, 2 out]
                  n641 = property on="E2" class="Bool (strict)"("Position"=T3 {"Left"=876, "Top"=420} ("Position 28")) -> ()  [unwired: 2 in, 2 out]
                  n642 = property on="E1" class="Bool (strict)"("Position"=T3 {"Left"=876, "Top"=396} ("Position 27")) -> ()  [unwired: 2 in, 2 out]
                  n643 = property on="W1" class="Bool (strict)"("Position"=T3 {"Left"=840, "Top"=396} ("Position 19")) -> ()  [unwired: 2 in, 2 out]
                  n644 = property on="W2" class="Bool (strict)"("Position"=T3 {"Left"=840, "Top"=420} ("Position 20")) -> ()  [unwired: 2 in, 2 out]
                  n645 = property on="Pause 2" class="Bool (strict)"("Position"=T3 {"Left"=1068, "Top"=456}) -> ()  [unwired: 2 in, 2 out]
                  n646 = property on="Pause 1" class="Bool (strict)"("Position"=T3 {"Left"=1068, "Top"=432} ("Position 2")) -> ()  [unwired: 2 in, 2 out]
                  n647 = property on="TL 3" class="Bool (strict)"("Position"=T3 {"Left"=876, "Top"=204} ("Position 6")) -> ()  [unwired: 2 in, 2 out]
                  n648 = property on="TL 2" class="Bool (strict)"("Position"=T3 {"Left"=804, "Top"=235} ("Position 5")) -> ()  [unwired: 2 in, 2 out]
                  n649 = property on="CL 3" class="Bool (strict)"("Position"=T3 {"Left"=876, "Top"=180} ("Position 8")) -> ()  [unwired: 2 in, 2 out]
                  n650 = property on="CL 2" class="Bool (strict)"("Position"=T3 {"Left"=804, "Top"=259} ("Position 7")) -> ()  [unwired: 2 in, 2 out]
                  n651 = property on="BL 3" class="Bool (strict)"("Position"=T3 {"Left"=876, "Top"=156} ("Position 10")) -> ()  [unwired: 2 in, 2 out]
                  n652 = property on="BL 2" class="Bool (strict)"("Position"=T3 {"Left"=804, "Top"=283} ("Position 9")) -> ()  [unwired: 2 in, 2 out]
                  n653 = property on="S1" class="Bool (strict)"("Position"=T3 {"Left"=936, "Top"=384} ("Position 11")) -> ()  [unwired: 2 in, 2 out]
                  n654 = property on="S2" class="Bool (strict)"("Position"=T3 {"Left"=936, "Top"=432} ("Position 12")) -> ()  [unwired: 2 in, 2 out]
                  n655 = property on="TM 3" class="Bool (strict)"("Position"=T3 {"Left"=840, "Top"=204} ("Position 14")) -> ()  [unwired: 2 in, 2 out]
                  n656 = property on="TM 2" class="Bool (strict)"("Position"=T3 {"Left"=840, "Top"=235} ("Position 13")) -> ()  [unwired: 2 in, 2 out]
                  n657 = property on="CM 3" class="Bool (strict)"("Position"=T3 {"Left"=840, "Top"=180} ("Position 16")) -> ()  [unwired: 2 in, 2 out]
                  n658 = property on="CM 2" class="Bool (strict)"("Position"=T3 {"Left"=840, "Top"=259} ("Position 15")) -> ()  [unwired: 2 in, 2 out]
                  n659 = property on="BM 3" class="Bool (strict)"("Position"=T3 {"Left"=840, "Top"=156} ("Position 18")) -> ()  [unwired: 2 in, 2 out]
                  n660 = property on="BM 2" class="Bool (strict)"("Position"=T3 {"Left"=840, "Top"=283} ("Position 17")) -> ()  [unwired: 2 in, 2 out]
                  n661 = property on="TR 3" class="Bool (strict)"("Position"=T3 {"Left"=804, "Top"=204} ("Position 22")) -> ()  [unwired: 2 in, 2 out]
                  n662 = property on="TR 2" class="Bool (strict)"("Position"=T3 {"Left"=876, "Top"=235} ("Position 21")) -> ()  [unwired: 2 in, 2 out]
                  n663 = property on="CR  3" class="Bool (strict)"("Position"=T3 {"Left"=804, "Top"=180} ("Position 24")) -> ()  [unwired: 2 in, 2 out]
                  n664 = property on="CR  2" class="Bool (strict)"("Position"=T3 {"Left"=876, "Top"=259} ("Position 23")) -> ()  [unwired: 2 in, 2 out]
                  n665 = property on="BR 3" class="Bool (strict)"("Position"=T3 {"Left"=804, "Top"=156} ("Position 26")) -> ()  [unwired: 2 in, 2 out]
                  n666 = property on="BR 2" class="Bool (strict)"("Position"=T3 {"Left"=876, "Top"=283} ("Position 25")) -> ()  [unwired: 2 in, 2 out]
                }
              }
              n667 = Increment(x="Progress...") -> (x+1=w1049:i32)
              n668 = call "IMAQ AVI Read Frame"("error in (no error)"=w1041, "Frame Number"=w1049, "Image"=w1042, "Avi Refnum"=w1048) -> ("Image Out"=w1021:T1)  [unwired: 4 in, 3 out]
              n669 = call "IMAQ Resample"("X Resolution"=680, "Y Resolution"=520, "error in (no error)"=w1020, "Image Dst"=w1019, "Image Src"=w1021) -> ("Image Dst Out"=w1022:T1)  [unwired: 5 in, 1 out]
              n670 = local read "F_frame"() -> (w1053:u32)
              n671 = Add(x=9, y=w1049) -> (x+y=w1052:i32)
              n672 = local write "Video"(w1022) -> ()
              n673 = Less Or Equal?(x=w1053, y=w1052) -> (x <= y?=w1030:bool)
              n674 = local read "framesPerSecond"() -> (w1025:u32)
              n675 = Select(t=w1052, s="fast forward", f=w1049) -> (s? t:f=w1029:i32)
              n676 = Select(t="Progress...", s=w1030, f=w1029) -> (s? t:f=w1027:i32)
              n677 = Divide(x=1000.0, y="playback speed") -> (x/y=w1056:dbl)
              n678 = Divide(x=w1056, y=w1025) -> (x/y=w1024:dbl)
              n679 = local write "Progress..."(w1027) -> ()
              n680 = Wait (ms)(milliseconds to wait=w1024) -> ()  [unwired: 1 out]
              n681 = Compound Arithmetic op=OR("Pause 1", "Pause 2", "Pause 3") -> (w1051:bool)
              n682 = case shown="True" w1051 {
                tunnel: w1049 -> [w1132 w1212]
                tunnel: [w1131 w1197] -> w1050
                tunnel: w1049 -> [_ w1215]
                tunnel: w1048 -> [w1129 w1214]
                tunnel: [w1129 w1211] -> w1047
                tunnel: "Pause 1" -> [_ w1210]
                tunnel: "Pause 2" -> [_ w1209]
                tunnel: w1024 -> [_ w1205]
                frame #0 {
                  n683 = local read "W1"() -> (w1128:bool)
                  n684 = local read "W2"() -> (w1126:bool)
                  n685 = local read "E1"() -> (w1127:bool)
                  n686 = local read "E2"() -> (w1125:bool)
                  n687 = Or(x=w1128, y=w1127) -> (x .or. y?=w1124:bool)
                  n688 = Or(x=w1126, y=w1125) -> (x .or. y?=w1123:bool)
                  n689 = Boolean To (0,1)(Boolean=w1124) -> (0, 1=w1121:i16)
                  n690 = Select(t=2.0, s=w1123, f=w1121) -> (s? t:f=w1120:dbl)
                  n691 = case shown="0, Default" w1120 {
                    tunnel: w1132 -> [_ _ _]
                    tunnel: [w1135 w1164 w1167] -> w1131
                    tunnel: [FALSE FALSE FALSE] -> w1130
                    frame #0 {
                      w1133 = FALSE ("4 6")
                      n692 = local write "1 6"(w1133) -> ()
                      n693 = local write "2 6"(w1133) -> ()
                      n694 = local write "3 6"(w1133) -> ()
                      n695 = local write "4 6"(w1133) -> ()
                      n696 = local write "5 6"(w1133) -> ()
                      n697 = local write "6 6"(w1133) -> ()
                      n698 = local write "7 6"(w1133) -> ()
                      n699 = local write "8 6"(w1133) -> ()
                      n700 = local write "1 5"(w1133) -> ()
                      n701 = local write "2 5"(w1133) -> ()
                      n702 = local write "3 5"(w1133) -> ()
                      n703 = local write "4 5"(w1133) -> ()
                      n704 = local write "5 5"(w1133) -> ()
                      n705 = local write "6 5"(w1133) -> ()
                      n706 = local write "7 5"(w1133) -> ()
                      n707 = local write "8 5"(w1133) -> ()
                      n708 = local write "1 4"(w1133) -> ()
                      n709 = local write "2 4"(w1133) -> ()
                      n710 = local write "3 4"(w1133) -> ()
                      n711 = local write "4 4"(w1133) -> ()
                      n712 = local write "5 4"(w1133) -> ()
                      n713 = local write "6 4"(w1133) -> ()
                      n714 = local write "7 4"(w1133) -> ()
                      n715 = local write "8 4"(w1133) -> ()
                      n716 = local write "1 3"(w1133) -> ()
                      n717 = local write "2 3"(w1133) -> ()
                      n718 = local write "3 3"(w1133) -> ()
                      n719 = local write "4 3"(w1133) -> ()
                      n720 = local write "5 3"(w1133) -> ()
                      n721 = local write "6 3"(w1133) -> ()
                      n722 = local write "7 3"(w1133) -> ()
                      n723 = local write "8 3"(w1133) -> ()
                      n724 = local write "1 2"(w1133) -> ()
                      n725 = local write "2 2"(w1133) -> ()
                      n726 = local write "3 2"(w1133) -> ()
                      n727 = local write "4 2"(w1133) -> ()
                      n728 = local write "5 2"(w1133) -> ()
                      n729 = local write "6 2"(w1133) -> ()
                      n730 = local write "7 2"(w1133) -> ()
                      n731 = local write "8 2"(w1133) -> ()
                      n732 = local write "1"(w1133) -> ()
                      n733 = local write "2"(w1133) -> ()
                      n734 = local write "3"(w1133) -> ()
                      n735 = local write "4"(w1133) -> ()
                      n736 = local write "5"(w1133) -> ()
                      n737 = local write "6"(w1133) -> ()
                      n738 = local write "7"(w1133) -> ()
                      n739 = local write "8"(w1133) -> ()
                      n740 = local write "BL 3"(w1133) -> ()
                      n741 = local write "BL 2"(w1133) -> ()
                      n742 = local write "BM 3"(w1133) -> ()
                      n743 = local write "BM 2"(w1133) -> ()
                      n744 = local write "BR 2"(w1133) -> ()
                      n745 = local write "BR 3"(w1133) -> ()
                      n746 = local write "W1"(w1133) -> ()
                      n747 = local write "W2"(w1133) -> ()
                      n748 = local write "E1"(w1133) -> ()
                      n749 = local write "E2"(w1133) -> ()
                      n750 = local write "TL 3"(w1133) -> ()
                      n751 = local write "TL 2"(w1133) -> ()
                      n752 = local write "TM 2"(w1133) -> ()
                      n753 = local write "TM 3"(w1133) -> ()
                      n754 = local write "TR 2"(w1133) -> ()
                      n755 = local write "TR 3"(w1133) -> ()
                      n756 = local write "S1"(w1133) -> ()
                      n757 = local write "S2"(w1133) -> ()
                      n758 = local write "1"(w1133) -> ()
                      n759 = local write "2"(w1133) -> ()
                      n760 = local write "3"(w1133) -> ()
                      n761 = local write "4"(w1133) -> ()
                      n762 = local write "CL 3"(w1133) -> ()
                      n763 = local write "CL 2"(w1133) -> ()
                      n764 = local write "CM 2"(w1133) -> ()
                      n765 = local write "CM 3"(w1133) -> ()
                      n766 = local write "CR  2"(w1133) -> ()
                      n767 = local write "CR  3"(w1133) -> ()
                      n768 = local read "coding"() -> (w1135:i32[][])
                    }
                    frame #1 {
                      n769 = local read "W1"() -> (w1158:bool)
                      n770 = local read "W2"() -> (w1159:bool)
                      n771 = local read "E1"() -> (w1160:bool)
                      n772 = local read "E2"() -> (w1161:bool)
                      n773 = Boolean To (0,1)(Boolean=w1158) -> (0, 1=w1150:i16)
                      n774 = Boolean To (0,1)(Boolean=w1159) -> (0, 1=w1149:i16)
                      n775 = Boolean To (0,1)(Boolean=w1160) -> (0, 1=w1144:i16)
                      n776 = Boolean To (0,1)(Boolean=w1161) -> (0, 1=w1143:i16)
                      n777 = Or(x=w1158, y=w1161) -> (x .or. y?=w1157:bool)
                      n778 = Or(x=w1159, y=w1160) -> (x .or. y?=w1156:bool)
                      n779 = local read "P2"() -> (w1136:i32)
                      n780 = local read "P1"() -> (w1162:i32)
                      n781 = Increment(x=w1162) -> (x+1=w1155:i32)
                      n782 = Increment(x=w1136) -> (x+1=w1154:i32)
                      n783 = Select(t=w1154, s=w1156, f=w1136) -> (s? t:f=w1137:i32)
                      n784 = Select(t=w1155, s=w1157, f=w1162) -> (s? t:f=w1139:i32)
                      n785 = Boolean To (0,1)(Boolean=w1157) -> (0, 1=w1142:i16)
                      n786 = Boolean To (0,1)(Boolean=w1156) -> (0, 1=w1141:i16)
                      n787 = local write "P1"(w1139) -> ()
                      n788 = local write "P2"(w1137) -> ()
                      n789 = local read "p1code"() -> (w1152:i32)
                      n790 = local read "coding"() -> (w1163:i32[][])
                      n791 = Replace Array Subset(array=w1163, new element #1=w1150, index (row) #1=w1152, index (col) #1=23 ("disabled index (col)"), new element #2=w1149, index (row) #2=w1152, index (col) #2=24 ("disabled index (col)"), new element #3=w1144, index (row) #3=w1152, index (col) #3=25 ("disabled index (col)"), new element #4=w1143, index (row) #4=w1152, index (col) #4=26 ("disabled index (col)"), new element #5=w1142, index (row) #5=w1152, index (col) #5=27 ("disabled index (col)"), new element #6=w1141, index (row) #6=w1152, index (col) #6=28 ("disabled index (col)"), new element #7=w1139, index (row) #7=w1152, index (col) #7=29 ("disabled index (col)"), new element #8=w1137, index (row) #8=w1152, index (col) #8=30 ("disabled index (col)")) -> (w1164:i32[][])
                      n792 = local write "coding"(w1164) -> ()
                    }
                    frame #2 {
                      n793 = local read "W1"() -> (w1190:bool)
                      n794 = local read "W2"() -> (w1191:bool)
                      n795 = local read "E1"() -> (w1192:bool)
                      n796 = local read "E2"() -> (w1193:bool)
                      n797 = Boolean To (0,1)(Boolean=w1190) -> (0, 1=w1183:i16)
                      n798 = Boolean To (0,1)(Boolean=w1191) -> (0, 1=w1182:i16)
                      n799 = Boolean To (0,1)(Boolean=w1192) -> (0, 1=w1177:i16)
                      n800 = Boolean To (0,1)(Boolean=w1193) -> (0, 1=w1176:i16)
                      n801 = Or(x=w1190, y=w1193) -> (x .or. y?=w1189:bool)
                      n802 = Or(x=w1191, y=w1192) -> (x .or. y?=w1188:bool)
                      n803 = local read "P2"() -> (w1166:i32)
                      n804 = local read "P1"() -> (w1194:i32)
                      n805 = Increment(x=w1194) -> (x+1=w1187:i32)
                      n806 = Increment(x=w1166) -> (x+1=w1186:i32)
                      n807 = Select(t=w1186, s=w1188, f=w1166) -> (s? t:f=w1170:i32)
                      n808 = Select(t=w1187, s=w1189, f=w1194) -> (s? t:f=w1172:i32)
                      n809 = Boolean To (0,1)(Boolean=w1189) -> (0, 1=w1175:i16)
                      n810 = Boolean To (0,1)(Boolean=w1188) -> (0, 1=w1174:i16)
                      n811 = local write "P1"(w1172) -> ()
                      n812 = local write "P2"(w1170) -> ()
                      n813 = local read "p2code"() -> (w1168:i32)
                      n814 = local read "coding"() -> (w1195:i32[][])
                      n815 = Replace Array Subset(array=w1195, new element #1=w1183, index (row) #1=w1168, index (col) #1=23 ("disabled index (col)"), new element #2=w1182, index (row) #2=w1168, index (col) #2=24 ("disabled index (col)"), new element #3=w1177, index (row) #3=w1168, index (col) #3=25 ("disabled index (col)"), new element #4=w1176, index (row) #4=w1168, index (col) #4=26 ("disabled index (col)"), new element #5=w1175, index (row) #5=w1168, index (col) #5=27 ("disabled index (col)"), new element #6=w1174, index (row) #6=w1168, index (col) #6=28 ("disabled index (col)"), new element #7=w1172, index (row) #7=w1168, index (col) #7=29 ("disabled index (col)"), new element #8=w1170, index (row) #8=w1168, index (col) #8=30 ("disabled index (col)")) -> (w1167:i32[][])
                      n816 = local write "coding"(w1167) -> ()
                    }
                  }
                  n817 = local write "W1"(w1130) -> ()
                  n818 = local write "W2"(w1130) -> ()
                  n819 = local write "E1"(w1130) -> ()
                  n820 = local write "E2"(w1130) -> ()
                }
                frame #1 {
                  n821 = stacked-sequence {
                    tunnel: [_ w1307 _ _ _ _ _ _] -> w1213
                    tunnel: [_ w1306 _ _ _ _ _ _] -> w1252
                    tunnel: [_ w1305 _ _ _ _ _ _] -> w1251
                    tunnel: [_ w1304 _ _ _ _ _ _] -> w1250
                    tunnel: [_ w1303 _ _ _ _ _ _] -> w1249
                    tunnel: [_ w1302 _ _ _ _ _ _] -> w1248
                    tunnel: [_ w1301 _ _ _ _ _ _] -> w1247
                    tunnel: [_ w1300 _ _ _ _ _ _] -> w1241
                    tunnel: [_ w1299 _ _ _ _ _ _] -> w1246
                    tunnel: [_ _ _ w1377 _ _ _ _] -> w1245
                    tunnel: [_ _ _ w1376 _ _ _ _] -> w1244
                    tunnel: [_ _ _ w1374 _ _ _ _] -> w1243
                    tunnel: [_ _ _ _ w1474 _ _ _] -> w1242
                    tunnel: [_ _ _ _ w1471 _ _ _] -> w1240
                    tunnel: [_ _ _ _ w1438 _ _ _] -> w1239
                    tunnel: [_ _ _ _ w1437 _ _ _] -> w1238
                    tunnel: [_ _ _ _ w1436 _ _ _] -> w1237
                    tunnel: [_ _ _ _ w1435 _ _ _] -> w1236
                    tunnel: [_ _ _ _ w1434 _ _ _] -> w1235
                    tunnel: [_ _ _ _ w1433 _ _ _] -> w1234
                    tunnel: [_ _ _ _ w1432 _ _ _] -> w1233
                    tunnel: [_ _ _ _ w1431 _ _ _] -> w1232
                    tunnel: [_ _ _ _ _ _ w1559 _] -> w1231
                    tunnel: [_ _ _ _ _ _ w1559 _] -> w1230
                    tunnel: [_ _ _ _ _ _ w1559 _] -> w1229
                    tunnel: [_ _ _ _ _ _ w1559 _] -> w1228
                    tunnel: [_ _ _ _ _ _ w1559 _] -> w1227
                    tunnel: [_ _ _ _ _ _ w1559 _] -> w1226
                    tunnel: [_ _ _ _ _ _ w1559 _] -> w1225
                    tunnel: [_ _ _ _ _ _ w1559 _] -> w1224
                    tunnel: [_ _ _ _ _ _ w1565 _] -> w1223
                    tunnel: [_ _ _ _ _ _ w1564 _] -> w1222
                    tunnel: [_ _ _ _ _ _ w1563 _] -> w1221
                    tunnel: [_ _ _ _ _ _ w1562 _] -> w1220
                    tunnel: [_ _ _ _ _ _ w1561 _] -> w1219
                    tunnel: [_ _ _ _ _ _ w1560 _] -> w1218
                    tunnel: [_ _ w1345 _ _ _ _ _] -> w1217
                    tunnel: [_ _ w1344 _ _ _ _ _] -> w1216
                    tunnel: w1215 -> [w1265 _ _ _ _ _ _ _]
                    tunnel: w1214 -> [w1264 _ _ _ _ _ _ _]
                    tunnel: [w1263 _ _ _ _ _ _ _] -> w1211
                    tunnel: [_ _ _ _ _ _ _ w1572] -> w1198
                    tunnel: w1210 -> [_ _ w1343 _ _ _ _ _]
                    tunnel: w1209 -> [_ _ w1342 _ _ _ _ _]
                    tunnel: w1205 -> [w1258 _ _ _ _ _ _ _]
                    tunnel: [w1257 _ _ _ _ _ _ _] -> w1196
                    frame #0 {
                      w1255 = T4 4 items=["Grayscale (U8)", "Grayscale (I16)", "Grayscale (SGL)", "Complex (CSG)", "RGB (U32)", "HSL (U32)", "RGB (U64)"] ("Image Type")
                      w1261 = T4 4 items=["Grayscale (U8)", "Grayscale (I16)", "Grayscale (SGL)", "Complex (CSG)", "RGB (U32)", "HSL (U32)", "RGB (U64)"] ("Image Type")
                      n822 = while {
                        tunnel: [FALSE] -> w1262
                        stop <- w1292 continue-if-true
                        n823 = local read "Pause 3"() -> (w1289:bool)
                        n824 = local read "Pause 1"() -> (w1290:bool)
                        n825 = local read "Pause 2"() -> (w1293:bool)
                        n826 = local read "coding"() -> (w1284:i32[][])
                        n827 = Compound Arithmetic op=OR(w1289, w1290, w1293) -> (w1292:bool)
                        n828 = Index Array(array=w1284, index (col)=0 ("disabled index (col)")) -> (element=w1287:i32[])  [unwired: 1 in]
                        n829 = Array Max & Min(array=w1287) -> (max value=w1286:i32, max index (indices)=w1283:i32)  [unwired: 2 out]
                        n830 = call "Time Delay4"("Delay Time (s)"=0.01) -> ()  [unwired: 10 in, 1 out]
                        n831 = case shown="True" "UNDO" {
                          selector: "UNDO" -> [w1294 _]
                          tunnel: w1284 -> [_ w1298]
                          tunnel: w1283 -> [_ w1297]
                          tunnel: [w1294 FALSE] -> w1282
                          frame #0 {
                          }
                          frame #1 {
                            n832 = Delete From Array(array=w1298, index (row)=w1297) -> (array with subset deleted=w1296:i32[][])  [unwired: 2 in, 1 out]
                            n833 = local write "coding"(w1296) -> ()
                          }
                        }
                        n834 = local write "Last coded"(w1286) -> ()
                        n835 = local write "UNDO"(w1282) -> ()
                      }
                      n836 = call "IMAQ Create"("Image Name"="code3", "Image Type"=w1261) -> ("New Image"=w1257:T1, "error out"=w1259:errorcluster)  [unwired: 3 in]
                      n837 = call "IMAQ Create"("Image Name"="code3 2", "Image Type"=w1255) -> ("New Image"=w1254:T1, "error out"=w1253:errorcluster)  [unwired: 3 in]
                      n838 = for {
                        N: 25 -> [_]
                        tunnel: w1265 -> [w1279]
                        tunnel: w1264 -> [w1277]
                        tunnel: w1259 -> [w1276]
                        tunnel: w1257 -> [w1275]
                        tunnel: [w1274] -> w1263
                        tunnel: w1258 -> [w1273]
                        tunnel: w1254 -> [w1270]
                        tunnel: w1253 -> [w1269]
                        i -> [w1280]
                        n839 = Add(x=w1280, y=w1279) -> (x+y=w1278:i32)
                        n840 = call "IMAQ AVI Read Frame"("error in (no error)"=w1276, "Frame Number"=w1278, "Image"=w1275, "Avi Refnum"=w1277) -> ("Image Out"=w1268:T1, "Avi Refnum (duplicate)"=w1274:T5)  [unwired: 4 in, 2 out]
                        n841 = call "IMAQ Resample"("X Resolution"=680, "Y Resolution"=520, "error in (no error)"=w1269, "Image Dst"=w1270, "Image Src"=w1268) -> ("Image Dst Out"=w1267:T1)  [unwired: 5 in, 1 out]
                        n842 = Wait (ms)(milliseconds to wait=w1273) -> ()  [unwired: 1 out]
                        n843 = local write "Video"(w1267) -> ()
                      }
                      n844 = local write "Pause 1"(w1262) -> ()
                      n845 = local write "Pause 2"(w1262) -> ()
                      n846 = local write "Pause 3"(w1262) -> ()
                      n847 = local write "UNDO"(w1262) -> ()
                    }
                    frame #1 {
                      n848 = Or(x="TM 2", y="TM 3") -> (x .or. y?=w1315:bool)
                      n849 = Or(x="CL 3", y="CL 2") -> (x .or. y?=w1313:bool)
                      n850 = Or(x="CR  2", y="CR  3") -> (x .or. y?=w1311:bool)
                      n851 = Or(x="BM 3", y="BM 2") -> (x .or. y?=w1309:bool)
                      n852 = Boolean To (0,1)(Boolean=w1315) -> (0, 1=w1306:i16)
                      n853 = Boolean To (0,1)(Boolean=w1313) -> (0, 1=w1304:i16)
                      n854 = Boolean To (0,1)(Boolean=w1311) -> (0, 1=w1302:i16)
                      n855 = Boolean To (0,1)(Boolean=w1309) -> (0, 1=w1300:i16)
                      n856 = Or(x="TL 3", y="TL 2") -> (x .or. y?=w1316:bool)
                      n857 = Or(x="TR 2", y="TR 3") -> (x .or. y?=w1314:bool)
                      n858 = Or(x="CM 2", y="CM 3") -> (x .or. y?=w1312:bool)
                      n859 = Or(x="BL 3", y="BL 2") -> (x .or. y?=w1310:bool)
                      n860 = Or(x="BR 2", y="BR 3") -> (x .or. y?=w1308:bool)
                      n861 = Boolean To (0,1)(Boolean=w1316) -> (0, 1=w1307:i16)
                      n862 = Boolean To (0,1)(Boolean=w1314) -> (0, 1=w1305:i16)
                      n863 = Boolean To (0,1)(Boolean=w1312) -> (0, 1=w1303:i16)
                      n864 = Boolean To (0,1)(Boolean=w1310) -> (0, 1=w1301:i16)
                      n865 = Boolean To (0,1)(Boolean=w1308) -> (0, 1=w1299:i16)
                    }
                    frame #2 {
                      n866 = local read "S1"() -> (w1341:bool)
                      n867 = local read "S2"() -> (w1340:bool)
                      n868 = local read "CM 3"() -> (w1369:bool)
                      n869 = local read "TM 3"() -> (w1370:bool)
                      n870 = local read "BM 3"() -> (w1368:bool)
                      n871 = local read "CR  3"() -> (w1365:bool)
                      n872 = local read "CL 3"() -> (w1371:bool)
                      n873 = local read "BR 3"() -> (w1367:bool)
                      n874 = local read "TR 3"() -> (w1366:bool)
                      n875 = local read "BL 3"() -> (w1373:bool)
                      n876 = local read "TL 3"() -> (w1372:bool)
                      n877 = Or(x=w1341, y=w1340) -> (x .or. y?=w1336:bool)
                      n878 = Compound Arithmetic op=OR(w1373, w1372, w1371, w1370, w1369, w1368, w1367, w1366, w1365) -> (w1347:bool)
                      "P1 position" <- w1347
                      n879 = Or(x=w1347, y=w1343) -> (x .or. y?=w1338:bool)
                      n880 = Or(x=w1338, y=w1336) -> (x .or. y?=w1339:bool)
                      n881 = local read "coding"() -> (w1355:i32[][])
                      n882 = local read "CM 2"() -> (w1361:bool)
                      n883 = local read "TM 2"() -> (w1362:bool)
                      n884 = local read "BM 2"() -> (w1360:bool)
                      n885 = local read "CR  2"() -> (w1359:bool)
                      n886 = local read "CL 2"() -> (w1356:bool)
                      n887 = local read "TR 2"() -> (w1358:bool)
                      n888 = local read "BR 2"() -> (w1357:bool)
                      n889 = local read "BL 2"() -> (w1364:bool)
                      n890 = local read "TL 2"() -> (w1363:bool)
                      n891 = Boolean To (0,1)(Boolean=w1339) -> (0, 1=w1345:i16)
                      n892 = Array Size(array=w1355) -> (size(s)=w1354:i32[])
                      n893 = Compound Arithmetic op=OR(w1364, w1363, w1356, w1362, w1361, w1360, w1359, w1358, w1357) -> (w1346:bool)
                      "P2 position" <- w1346
                      n894 = local read "p1code"() -> (w1351:i32)
                      n895 = Index Array(array=w1354, index=0) -> (element=w1349:i32)
                      n896 = Or(x=w1346, y=w1342) -> (x .or. y?=w1337:bool)
                      n897 = Or(x=w1337, y=w1336) -> (x .or. y?=w1335:bool)
                      n898 = Select(t=w1349, s=w1339, f=w1351) -> (s? t:f=→"p1code":i32)
                      n899 = local read "p2code"() -> (w1348:i32)
                      n900 = Select(t=w1349, s=w1335, f=w1348) -> (s? t:f=→"p2code":i32)
                      n901 = Boolean To (0,1)(Boolean=w1335) -> (0, 1=w1344:i16)
                    }
                    frame #3 {
                      n902 = Build Array("1", "2", "3", "4", "5", "6", "7", "8", "1 2", "2 2", "3 2", "4 2", "5 2", "6 2", "7 2", "8 2") -> (w1398:bool[])
                      "FH" <- w1398
                      n903 = Or Array Elements(Boolean array=w1398) -> (logical OR=w1379:bool)
                      n904 = Boolean To (0,1)(Boolean=w1379) -> (0, 1=w1377:i16)
                      n905 = Build Array("1 3", "2 3", "3 3", "4 3", "5 3", "6 3", "7 3", "8 3", "1 4", "2 4", "3 4", "4 4", "5 4", "6 4", "7 4", "8 4") -> (w1381:bool[])
                      "BH" <- w1381
                      n906 = Or Array Elements(Boolean array=w1381) -> (logical OR=w1378:bool)
                      n907 = Boolean To (0,1)(Boolean=w1378) -> (0, 1=w1376:i16)
                      n908 = Build Array("1 5", "2 5", "3 5", "4 5", "5 5", "6 5", "7 5", "8 5", "1 6", "2 6", "3 6", "4 6", "5 6", "6 6", "7 6", "8 6") -> (w1380:bool[])
                      "OH" <- w1380
                      n909 = Or Array Elements(Boolean array=w1380) -> (logical OR=w1375:bool)
                      n910 = Boolean To (0,1)(Boolean=w1375) -> (0, 1=w1374:i16)
                    }
                    frame #4 {
                      w1479 = 8 ("index")
                      n911 = local read "OH"() -> (w1468:bool[])
                      n912 = local read "BH"() -> (w1469:bool[])
                      n913 = local read "FH"() -> (w1470:bool[])
                      n914 = Split 1D Array(array=w1470, index=w1479) -> (first subarray=w1466:bool[], second subarray=w1467:bool[])
                      n915 = Split 1D Array(array=w1469, index=w1479) -> (first subarray=w1478:bool[], second subarray=w1476:bool[])
                      n916 = Split 1D Array(array=w1468, index=w1479) -> (first subarray=w1477:bool[], second subarray=w1475:bool[])
                      n917 = Build Array(w1466, w1478, w1477) -> (w1465:bool[][])
                      n918 = Build Array(w1467, w1476, w1475) -> (w1464:bool[][])
                      n919 = Or Array Elements(Boolean array=w1465) -> (logical OR=w1473:bool)
                      n920 = Or Array Elements(Boolean array=w1464) -> (logical OR=w1472:bool)
                      n921 = Insert Into Array(array=w1465, new element=w1464) -> (w1463:bool[][])  [unwired: 2 in]
                      n922 = Boolean To (0,1)(Boolean=w1473) -> (0, 1=w1474:i16)
                      n923 = Boolean To (0,1)(Boolean=w1472) -> (0, 1=w1471:i16)
                      n924 = Index Array(array=w1463, index (col) #1=3 ("disabled index (col)"), index (col) #2=4 ("index (col)"), index (col) #3=2 ("index (col)"), index (col) #4=1 ("index (col)"), index (col) #5=6 ("index (col)"), index (col) #6=5 ("index (col)"), index (col) #7=0 ("index (col)"), index (col) #8=7 ("index (col)")) -> (element #1=w1453:bool[], element #2=w1445:bool[], element #3=w1444:bool[], element #4=w1443:bool[], element #5=w1442:bool[], element #6=w1441:bool[], element #7=w1440:bool[], element #8=w1439:bool[])  [unwired: 8 in]
                      n925 = Or Array Elements(Boolean array=w1453) -> (logical OR=w1454:bool)
                      n926 = Or Array Elements(Boolean array=w1444) -> (logical OR=w1450:bool)
                      n927 = Or Array Elements(Boolean array=w1442) -> (logical OR=w1449:bool)
                      n928 = Or Array Elements(Boolean array=w1440) -> (logical OR=w1446:bool)
                      n929 = Or Array Elements(Boolean array=w1445) -> (logical OR=w1452:bool)
                      n930 = Or Array Elements(Boolean array=w1443) -> (logical OR=w1451:bool)
                      n931 = Or Array Elements(Boolean array=w1441) -> (logical OR=w1448:bool)
                      n932 = Or Array Elements(Boolean array=w1439) -> (logical OR=w1447:bool)
                      n933 = Boolean To (0,1)(Boolean=w1454) -> (0, 1=w1438:i16)
                      n934 = Boolean To (0,1)(Boolean=w1450) -> (0, 1=w1436:i16)
                      n935 = Boolean To (0,1)(Boolean=w1449) -> (0, 1=w1434:i16)
                      n936 = Boolean To (0,1)(Boolean=w1446) -> (0, 1=w1432:i16)
                      n937 = Boolean To (0,1)(Boolean=w1452) -> (0, 1=w1437:i16)
                      n938 = Boolean To (0,1)(Boolean=w1451) -> (0, 1=w1435:i16)
                      n939 = Boolean To (0,1)(Boolean=w1448) -> (0, 1=w1433:i16)
                      n940 = Boolean To (0,1)(Boolean=w1447) -> (0, 1=w1431:i16)
                    }
                    frame #5 {
                      n941 = local read "P2 position"() -> (w1494:bool)
                      n942 = local read "P1 position"() -> (w1490:bool)
                      n943 = local read "BH"() -> (w1488:bool[])
                      n944 = local read "OH"() -> (w1489:bool[])
                      n945 = local read "FH"() -> (w1487:bool[])
                      n946 = Or(x="W2", y="E2") -> (x .or. y?=w1498:bool)
                      n947 = Or(x="W1", y="E1") -> (x .or. y?=w1495:bool)
                      n948 = Or Array Elements(Boolean array=w1488) -> (logical OR=w1492:bool)
                      n949 = Or Array Elements(Boolean array=w1489) -> (logical OR=w1493:bool)
                      n950 = Or Array Elements(Boolean array=w1487) -> (logical OR=w1491:bool)
                      n951 = Compound Arithmetic op=OR(w1490, w1491, w1492, w1493, w1494) -> (invert w1497:bool)
                      n952 = And(x=w1497, y=w1498) -> (x .and. y?=w1499:bool)
                      n953 = And(x=w1497, y=w1495) -> (x .and. y?=w1496:bool)
                      n954 = Boolean To (0,1)(Boolean=w1496) -> (0, 1=w1486:i16)
                      n955 = Select(t=2.0, s=w1499, f=w1486) -> (s? t:f=w1481:dbl)
                      n956 = case shown="0, Default" w1481 {
                        tunnel: [w1500 w1529 w1532] -> _
                        frame #0 {
                          n957 = local read "coding"() -> (w1500:i32[][])
                        }
                        frame #1 {
                          n958 = local read "W1"() -> (w1523:bool)
                          n959 = local read "W2"() -> (w1524:bool)
                          n960 = local read "P2"() -> (w1501:i32)
                          n961 = local read "E1"() -> (w1525:bool)
                          n962 = local read "E2"() -> (w1526:bool)
                          n963 = local read "P1"() -> (w1527:i32)
                          n964 = Increment(x=w1501) -> (x+1=w1519:i32)
                          n965 = Or(x=w1524, y=w1525) -> (x .or. y?=w1521:bool)
                          n966 = Increment(x=w1527) -> (x+1=w1520:i32)
                          n967 = Or(x=w1523, y=w1526) -> (x .or. y?=w1522:bool)
                          n968 = Boolean To (0,1)(Boolean=w1523) -> (0, 1=w1515:i16)
                          n969 = Boolean To (0,1)(Boolean=w1524) -> (0, 1=w1514:i16)
                          n970 = Boolean To (0,1)(Boolean=w1525) -> (0, 1=w1509:i16)
                          n971 = Boolean To (0,1)(Boolean=w1526) -> (0, 1=w1508:i16)
                          n972 = Select(t=w1519, s=w1521, f=w1501) -> (s? t:f=w1502:i32)
                          n973 = Select(t=w1520, s=w1522, f=w1527) -> (s? t:f=w1504:i32)
                          n974 = local read "p1code"() -> (w1517:i32)
                          n975 = local read "coding"() -> (w1528:i32[][])
                          n976 = Boolean To (0,1)(Boolean=w1522) -> (0, 1=w1507:i16)
                          n977 = Boolean To (0,1)(Boolean=w1521) -> (0, 1=w1506:i16)
                          n978 = local write "P1"(w1504) -> ()
                          n979 = local write "P2"(w1502) -> ()
                          n980 = Replace Array Subset(array=w1528, new element #1=w1515, index (row) #1=w1517, index (col) #1=23 ("disabled index (col)"), new element #2=w1514, index (row) #2=w1517, index (col) #2=24 ("disabled index (col)"), new element #3=w1509, index (row) #3=w1517, index (col) #3=25 ("disabled index (col)"), new element #4=w1508, index (row) #4=w1517, index (col) #4=26 ("disabled index (col)"), new element #5=w1507, index (row) #5=w1517, index (col) #5=27 ("disabled index (col)"), new element #6=w1506, index (row) #6=w1517, index (col) #6=28 ("disabled index (col)"), new element #7=w1504, index (row) #7=w1517, index (col) #7=29 ("disabled index (col)"), new element #8=w1502, index (row) #8=w1517, index (col) #8=30 ("disabled index (col)")) -> (w1529:i32[][])
                          n981 = local write "coding"(w1529) -> ()
                        }
                        frame #2 {
                          n982 = local read "W1"() -> (w1554:bool)
                          n983 = local read "W2"() -> (w1555:bool)
                          n984 = local read "E1"() -> (w1556:bool)
                          n985 = local read "E2"() -> (w1557:bool)
                          n986 = Increment(x="P1") -> (x+1=w1551:i32)
                          n987 = Boolean To (0,1)(Boolean=w1554) -> (0, 1=w1547:i16)
                          n988 = Boolean To (0,1)(Boolean=w1555) -> (0, 1=w1546:i16)
                          n989 = Boolean To (0,1)(Boolean=w1556) -> (0, 1=w1541:i16)
                          n990 = Boolean To (0,1)(Boolean=w1557) -> (0, 1=w1540:i16)
                          n991 = Or(x=w1554, y=w1557) -> (x .or. y?=w1553:bool)
                          n992 = Or(x=w1555, y=w1556) -> (x .or. y?=w1552:bool)
                          n993 = Increment(x="P2") -> (x+1=w1550:i32)
                          n994 = Select(t=w1550, s=w1552, f="P2") -> (s? t:f=w1534:i32)
                          n995 = Select(t=w1551, s=w1553, f="P1") -> (s? t:f=w1536:i32)
                          n996 = Boolean To (0,1)(Boolean=w1553) -> (0, 1=w1539:i16)
                          n997 = Boolean To (0,1)(Boolean=w1552) -> (0, 1=w1538:i16)
                          n998 = local read "p2code"() -> (w1533:i32)
                          n999 = local read "coding"() -> (w1558:i32[][])
                          n1000 = local write "P1"(w1536) -> ()
                          n1001 = Replace Array Subset(array=w1558, new element #1=w1547, index (row) #1=w1533, index (col) #1=23 ("disabled index (col)"), new element #2=w1546, index (row) #2=w1533, index (col) #2=24 ("disabled index (col)"), new element #3=w1541, index (row) #3=w1533, index (col) #3=25 ("disabled index (col)"), new element #4=w1540, index (row) #4=w1533, index (col) #4=26 ("disabled index (col)"), new element #5=w1539, index (row) #5=w1533, index (col) #5=27 ("disabled index (col)"), new element #6=w1538, index (row) #6=w1533, index (col) #6=28 ("disabled index (col)"), new element #7=w1536, index (row) #7=w1533, index (col) #7=29 ("disabled index (col)"), new element #8=w1534, index (row) #8=w1533, index (col) #8=30 ("disabled index (col)")) -> (w1532:i32[][])
                          n1002 = local write "P2"(w1534) -> ()
                          n1003 = local write "coding"(w1532) -> ()
                        }
                      }
                    }
                    frame #6 {
                      w1559 = i16 0
                      n1004 = Boolean To (0,1)(Boolean="S1") -> (0, 1=w1565:i16)
                      n1005 = Boolean To (0,1)(Boolean="S2") -> (0, 1=w1564:i16)
                      n1006 = Boolean To (0,1)(Boolean="1") -> (0, 1=w1563:i16)
                      n1007 = Boolean To (0,1)(Boolean="2") -> (0, 1=w1562:i16)
                      n1008 = Boolean To (0,1)(Boolean="3") -> (0, 1=w1561:i16)
                      n1009 = Boolean To (0,1)(Boolean="4") -> (0, 1=w1560:i16)
                    }
                    frame #7 {
                      w1573 = FALSE ("4 6")
                      n1010 = local write "1 6"(w1573) -> ()
                      n1011 = local write "2 6"(w1573) -> ()
                      n1012 = local write "3 6"(w1573) -> ()
                      n1013 = local write "4 6"(w1573) -> ()
                      n1014 = local write "5 6"(w1573) -> ()
                      n1015 = local write "6 6"(w1573) -> ()
                      n1016 = local write "7 6"(w1573) -> ()
                      n1017 = local write "8 6"(w1573) -> ()
                      n1018 = local write "1 5"(w1573) -> ()
                      n1019 = local write "2 5"(w1573) -> ()
                      n1020 = local write "3 5"(w1573) -> ()
                      n1021 = local write "4 5"(w1573) -> ()
                      n1022 = local write "5 5"(w1573) -> ()
                      n1023 = local write "6 5"(w1573) -> ()
                      n1024 = local write "7 5"(w1573) -> ()
                      n1025 = local write "8 5"(w1573) -> ()
                      n1026 = local write "1 4"(w1573) -> ()
                      n1027 = local write "2 4"(w1573) -> ()
                      n1028 = local write "3 4"(w1573) -> ()
                      n1029 = local write "4 4"(w1573) -> ()
                      n1030 = local write "5 4"(w1573) -> ()
                      n1031 = local write "6 4"(w1573) -> ()
                      n1032 = local write "7 4"(w1573) -> ()
                      n1033 = local write "8 4"(w1573) -> ()
                      n1034 = local write "1 3"(w1573) -> ()
                      n1035 = local write "2 3"(w1573) -> ()
                      n1036 = local write "3 3"(w1573) -> ()
                      n1037 = local write "4 3"(w1573) -> ()
                      n1038 = local write "5 3"(w1573) -> ()
                      n1039 = local write "6 3"(w1573) -> ()
                      n1040 = local write "7 3"(w1573) -> ()
                      n1041 = local write "8 3"(w1573) -> ()
                      n1042 = local write "1 2"(w1573) -> ()
                      n1043 = local write "2 2"(w1573) -> ()
                      n1044 = local write "3 2"(w1573) -> ()
                      n1045 = local write "4 2"(w1573) -> ()
                      n1046 = local write "5 2"(w1573) -> ()
                      n1047 = local write "6 2"(w1573) -> ()
                      n1048 = local write "7 2"(w1573) -> ()
                      n1049 = local write "8 2"(w1573) -> ()
                      n1050 = local write "1"(w1573) -> ()
                      n1051 = local write "2"(w1573) -> ()
                      n1052 = local write "3"(w1573) -> ()
                      n1053 = local write "4"(w1573) -> ()
                      n1054 = local write "5"(w1573) -> ()
                      n1055 = local write "6"(w1573) -> ()
                      n1056 = local write "7"(w1573) -> ()
                      n1057 = local write "8"(w1573) -> ()
                      n1058 = local write "BL 3"(w1573) -> ()
                      n1059 = local write "BL 2"(w1573) -> ()
                      n1060 = local write "BM 3"(w1573) -> ()
                      n1061 = local write "BM 2"(w1573) -> ()
                      n1062 = local write "BR 2"(w1573) -> ()
                      n1063 = local write "BR 3"(w1573) -> ()
                      n1064 = local write "W1"(w1573) -> ()
                      n1065 = local write "W2"(w1573) -> ()
                      n1066 = local write "E1"(w1573) -> ()
                      n1067 = local write "E2"(w1573) -> ()
                      n1068 = local write "TL 3"(w1573) -> ()
                      n1069 = local write "TL 2"(w1573) -> ()
                      n1070 = local write "TM 2"(w1573) -> ()
                      n1071 = local write "TM 3"(w1573) -> ()
                      n1072 = local write "TR 2"(w1573) -> ()
                      n1073 = local write "TR 3"(w1573) -> ()
                      n1074 = local write "S1"(w1573) -> ()
                      n1075 = local write "S2"(w1573) -> ()
                      n1076 = local write "1"(w1573) -> ()
                      n1077 = local write "2"(w1573) -> ()
                      n1078 = local write "3"(w1573) -> ()
                      n1079 = local write "4"(w1573) -> ()
                      n1080 = local read "coding"() -> (w1572:i32[][])
                      n1081 = local write "CL 3"(w1573) -> ()
                      n1082 = local write "CL 2"(w1573) -> ()
                      n1083 = local write "CM 2"(w1573) -> ()
                      n1084 = local write "CM 3"(w1573) -> ()
                      n1085 = local write "CR  2"(w1573) -> ()
                      n1086 = local write "CR  3"(w1573) -> ()
                    }
                  }
                  n1087 = call "IMAQ Dispose"("Image"=w1196) -> ()  [unwired: 5 in, 1 out]
                  n1088 = Build Array(w1212, w1213, w1252, w1251, w1250, w1249, w1248, w1247, w1241, w1246, w1245, w1244, w1243, w1242, w1240, w1239, w1238, w1237, w1236, w1235, w1234, w1233, w1232, w1231, w1230, w1229, w1228, w1227, w1226, w1225, w1224, w1223, w1222, w1221, w1220, w1219, w1218, w1217, w1216) -> (w1204:i32[])
                  n1089 = Delete From Array(array=w1204, index=0) -> (array with subset deleted=w1202:i32[])  [unwired: 1 in, 1 out]
                  n1090 = Insert Into Array(array=w1198, new element=w1204) -> (w1199:i32[][])  [unwired: 2 in]
                  n1091 = Array Max & Min(array=w1202) -> (max value=w1201:i32)  [unwired: 3 out]
                  n1092 = Equal To 0?(x=w1201) -> (x = 0?=w1200:bool)
                  n1093 = Select(t=w1198, s=w1200, f=w1199) -> (s? t:f=w1197:i32[][])
                  n1094 = Index Array(array=w1197, index (col)=0 ("disabled index (col)")) -> (element=w1206:i32[])  [unwired: 1 in]
                  n1095 = Array Max & Min(array=w1206) -> (max value=→"Last coded":i32)  [unwired: 3 out]
                  n1096 = local write "coding"(w1197) -> ()
                }
              }
              n1097 = case shown="True" "Stop and save" {
                tunnel: [FALSE ("T button?") w1061] -> w1026
                frame #0 {
                }
                frame #1 {
                  n1098 = Two Button Dialog(message="You are about to stop the notation process", 2:"Stop and Save" ("Left Button Text (\"Yes\")")) -> (T button?=w1061:bool)  [unwired: 1 in]
                }
              }
              n1099 = Strip Path(path="Save data") -> (stripped path=w1037:path)  [unwired: 1 out]
              n1100 = call <vilib>:"Get File Extension.vi"("file"="Save data") -> ("filename without extension"=w1040:string)  [unwired: 7 in, 3 out]
              n1101 = Path To String(path=w1037) -> (string=w1036:string)
              n1102 = Concatenate Strings(w1036, "\\" ("string"), w1040, "(BStAT DATA).xls" ("string")) -> (w1035:string)
              n1103 = String To Path(string=w1035) -> (path=w1032:path)
              n1104 = call <vilib>:"Check if File or Folder Exists.vi"("path"=w1032) -> ("file or folder exists?"=w1033:bool)  [unwired: 8 in, 2 out]
            }
            n1105 = local read "F_frame"() -> (w1001:u32)
            n1106 = local read "S_frame"() -> (w1000:u32)
            n1107 = property on="Progress..." class="Slide (strict)"("Scale.Maximum"=w1001, "Scale.Minimum"=w1000, "Visible"=w985) -> ()  [unwired: 2 in, 2 out]
            n1108 = Not(x=w985) -> (.not. x?=w986:bool)
            n1109 = property on="Drag control" class="Slide (strict)"("Visible"=w986) -> ()  [unwired: 2 in, 2 out]
            n1110 = Path to Array of Strings(0:w995) -> (2:w996:string[])  [unwired: 1 out]
            n1111 = Array Size(array=w996) -> (size(s)=w997:i32)
            n1112 = Decrement(x=w997) -> (x-1=w998:i32)
            n1113 = Index Array(array=w996, index=w998) -> (element=w994:string)
            n1114 = call "EVENTS(SubVI).vi"() -> ("Events"=w992:string)  [unwired: 1 in]
            n1115 = Concatenate Strings("avi file" ("string"), w991, w994, w991, w991, w992) -> (w993:string)
            n1116 = call "IMAQ AVI Close"("Avi Refnum"=w989) -> ()  [unwired: 10 in, 1 out]
            n1117 = case shown="False" w983 {
              tunnel: w984 -> [w1014 w1016]
              tunnel: w993 -> [w1011 _]
              tunnel: w982 -> [w1009 w1015]
              frame #0 {
                n1118 = Open/Create/Replace File(file path (use dialog)=w1009, operation (0:open)=T2."create") -> (refnum out=w1012:refnum<file>)  [unwired: 4 in, 2 out]
                n1119 = Write to Text File(file (use dialog)=w1012, text=w1011) -> (refnum out=w1008:refnum<file>)  [unwired: 2 in, 2 out]
                n1120 = Close File(refnum=w1008) -> (path=w1007:path)  [unwired: 1 in, 1 out]
                n1121 = call-poly <vilib>:"Write To Spreadsheet File.vi"("append to file? (new file:F)"=TRUE, "2D data"=w1014, "file path (dialog if empty)"=w1007) -> ()  [unwired: 5 in, 1 out]
              }
              frame #1 {
                n1122 = call-poly <vilib>:"Write To Spreadsheet File.vi"("append to file? (new file:F)"=TRUE, "2D data"=w1016, "file path (dialog if empty)"=w1015) -> ()  [unwired: 5 in, 1 out]
              }
            }
            n1123 = property on="playback speed" class="Slide (strict)"("Visible"=w988) -> ()  [unwired: 2 in, 2 out]
            n1124 = property on="Progress..." class="Slide (strict)"("Visible"=w988) -> ()  [unwired: 2 in, 2 out]
            n1125 = property on="UNDO" class="Bool (strict)"("Visible"=w988) -> ()  [unwired: 2 in, 2 out]
            n1126 = property on="Last coded" class="DigNum (strict)"("Visible"=w988) -> ()  [unwired: 2 in, 2 out]
            n1127 = property on="Last coded" class="DigNum (strict)"("Visible"=w987) -> ()  [unwired: 2 in, 2 out]
            n1128 = property on="UNDO" class="Bool (strict)"("Visible"=w987) -> ()  [unwired: 2 in, 2 out]
            n1129 = property on="playback speed" class="Slide (strict)"("Visible"=w987) -> ()  [unwired: 2 in, 2 out]
            "coding" <- i32[][] [] ("coding")
          }
        }
        "S_frame" <- w929
        "F_frame" <- w929
      }
    }
  }
